vi "CurlingRobotforSweepHOST.vi"() -> ()   [LabVIEW 2015]
uses:
  <vilib>/IEDriver/SPIandI2C/Host/I2C/I2C Host.lvlib
  <vilib>/rvi/interface/nirviCloseFPGA/nirviCloseFPGA.xnode
  <vilib>/rvi/interface/nirviOpenFPGA/nirviOpenFPGA.xnode
  <vilib>/Platform/TimedLoop/XDataNode/wakeup.ctl
  <vilib>/Platform/TimedLoop/XDataNode/XDNodeRunTimeDep.lvlib
  <vilib>/Platform/TimedLoop/XDataNode/nitl_modes.ctl
  <vilib>/Platform/TimedLoop/XDataNode/timing_clust.ctl
  <vilib>/Platform/TimedLoop/XDataNode/XDataNode.xnode
  <vilib>/rvi/interface/nirviReadWriteControl/nirviReadWriteControl.xnode
  <vilib>/rvi/errors/niLvFpgaAdjustHostInterfaceError.vi
  <vilib>/rvi/interface/Simulation/niFpgaSimulationCallBeginRW.vi
  <vilib>/Instr/_visa.llb/VISA Flush IO Buffer Mask.ctl
  <vilib>/rvi/interface/nirviMethod/nirviMethod.xnode
  <vilib>/FPGAPlugInAG/Dynamic/niLvFpga_Reset_Dynamic.vi
  <vilib>/FPGAPlugInAG/Dynamic/niLvFpga_Run_Dynamic.vi
  cRIO_sweeping/SBC/Labview_exp/cRIO_sweeping/FPGA Bitfiles/testcomm_FPGATarget_FPGAsweepingaccg_gPSmUup16AQ.lvbitx
  cRIO_sweeping/SBC/Labview_exp/cRIO_sweeping/FPGA_sweeping_acc_gyro_v2.vi
  <vilib>/FPGAPlugInAG/cRIO-9033/niLvFpga_Open_cRIO-9033.vi
  <vilib>/rvi/interface/common/dynamic/niFpgaDynamicAddResources.vi
  NiFpgaLv.dll
  <vilib>/Utility/error.llb/Error Cluster From Error Code.vi
  <vilib>/FPGAPlugInAG/Dynamic/niLvFpga_Close_Dynamic.vi
  <vilib>/Instr/_visa.llb/VISA Configure Serial Port (Instr).vi
panel:
  in  "AddStAng":dbl=-7.0
  in  "FileCreat":bool
  out "AutobackCmd":i16(graph)
  in  "yStop":dbl=0.3 format="%#_13g"
  in  "upperx":dbl=0.3
  in  "downx":dbl=0.1 format="%#_13g"
  in  "LImitX":dbl=0.3 format="%#_13g"
  out "SBCAutoback":dbl
  out "NowVel13":dbl=-4.456150742348873e-97
  out "Steer_Rear":dbl=2.887351226806641
  out "RearSteerCmd":dbl
  out "CompleteAutoback":bool
  out "AutobackVel":dbl
  out "AutobackOn":bool
  out "Tqoff_autoback":bool=TRUE
  out "Time_autoback":dbl
  out "SBCvariable":dbl(graph)=2.0
  out "SBC2mode":bool
  out "sum_y":dbl=-7.853981633974483e-05
  out "sum_x":dbl
  out "Steer_Left":dbl=2.190110778808594
  out "OldAng":dbl
  out "SinTx":dbl
  in  "TxHz":dbl=50.0
  out "VelRef":dbl
  out "AutoTimer":dbl=13.18
  out "SBCmode 2":dbl(graph)=2.0
  out "AngRer":dbl
  in  "file create":bool
  out "File create":i32=1
  in  "Stop Button":bool
  out "Numeric Control":i32
  in  "data iner":bool
  out "data innter":i32=60895
  out "SBCAngReset":bool
  in  "DriveStart":bool
  out "Timing":u32(graph)=1
  out "loopTime":u32=1
  out "Yawrate":dbl(graph)
  in  "TqOn(On)":bool=TRUE
  in  "VelRef_0(off)":bool
  out "SBCEncReset":bool
  out "NowAng":dbl=70.04209333359984
  out "Tq_cmd_Rear":dbl=25.392464820602626
  in  "AngRef_0(off)":bool
  out "Read Data 2":string="10 ,     286.690948   1 , 0, 0, \r\n"
  in  "0.1V/deg":dbl=0.105
  in  "SetSteer":bool
  in  "90/10\nRealAng":dbl=1.0
  in  "정지":bool
  out "send":i32=61118
  out "TCPRecieve":i32=58477
  in  "Ang_ref\n1v=10deg":dbl(slide)=-24.97797356828194 scale=-90.0..90.0
  in  "SBCOn":bool=TRUE
  in  "V_target":dbl(slide)=0.07826086956521738 scale=-3.0..3.0
  out "DOBOnSBC":bool
  out "AskSBC4ABS":bool
  out "AskSBC":i16
  out "SBCSteerEnable":bool=TRUE
  out "CompliteABS":bool
  out "SBCDriveEnable":bool
  in  "Stop 2":bool
  out "send2SBC1":i16
  out "send2SBC 2":dbl
  out "send2SBC 3":dbl=-7.853981633974483e-05
  out "send2SBC 4":dbl=-4.456150742348873e-97
  in  "SendDataOn":bool
  in  "AbsErrorCrit":dbl=0.1
  out "SetSteer2Ori(On)":bool=TRUE
  in  "Steer3OriAbs 3":dbl=242.0
  out "Steer3NowAbs":dbl
  in  "Steer2OriAbs 2":dbl=242.133
  out "Steer2NowAbs":dbl
  out "Steer1NowAbs 2":dbl
  in  "Steer1OriAbs":dbl=242.051
  out "AngCmdDOB":dbl=-0.0
  out "RearAngCmd":dbl=25.392464820602626
  in  "AngReset2nowAng":bool
  in  "PhiAngCUT":dbl=2.0 format="%#_13g"
  in  "NowConfigAngle":dbl
  out "bias per 0.5min":dbl=-0.05348200000000247
  out "YawAngFB":dbl=289.95791201460014
  in  "RearTqScale":dbl=0.8
  out "YR_FB":dbl
  out "Tq_cmd_L":dbl=25.406420183499797
  out "Tq_cmd_R":dbl=25.397816125171232
  out "Yawangle":dbl=286.690948
  out "steering 2":T1(graph)={"Steer_Left"=2.190110778808594, "Steer_Right"=2.457696533203125, "Steer_Rear"=2.887351226806641, "Steer_ang_ref[NoScale] "=0.0}
  out "Velocity":cluster{"V_target":dbl, "Vel_Robot":dbl}(graph)={"V_target"=0.0, "Vel_Robot"=-4.456150742348873e-97}
  in  "Kt_longi":dbl=0.12
  out "Steer_ang_ref[NoScale]":dbl
  out "Vel_cmd":dbl
  out "x_Rear":dbl=-7.853981633974483e-05
  out "x_L":dbl
  out "x_R":dbl=-2.617993877991494e-05
  in  "YR*_zero(off)":bool
  out "Yawangle*":dbl
  in  "PD_cut_rot 2":dbl=15.0
  in  "Kp_rot 3":dbl=0.0002
  in  "Kd_rot 4":dbl=7e-05
  out "Yaw angle":cluster{dbl, "y":dbl, "Yawangle*":dbl}(graph)={0.0, "y"=70.04209333359984, "Yawangle*"=0.0}
  out "Driving_Left":i64
  in  "탭 컨트롤":T2(tab)=enum."Communication"
  out "Pmod_YR":dbl=-0.0009155413138017853
  out "acc 3":cluster{i16, i16, i16}(graph)={-1, 1, 229}
  in  "Timeout (10 s) 3":u8=50
  out "error out 5":errorcluster
  in  "Address 4":u16=29 format="%.0x"
  in  "Port Number 4":u8
  in  "FPGA Clock (40 MHz) 4":u32=40000000
  in  "Clock Rate 4":u32=100000 caption="Clock Rate"
  in  "Address Type (7-bit) 4":enum16{"7-bit", "10-bit"}(ring)
  in  "Address":u16=105 format="%.0x"
  in  "Port Number":u8=2
  in  "FPGA Clock (40 MHz)":u32=40000000
  in  "Clock Rate":u32=100000
  in  "Timeout (10 s)":u8=50
  in  "Address Type (7-bit)":enum16{"7-bit", "10-bit"}(ring)
  out "error out 3":errorcluster
  out "Pmod_acc_z":dbl=0.94824016563147
  out "Check_FPGA_Delay_loop":i32=22187
  out "Check":bool=TRUE
  out "Gyro sensors":cluster{"Pmod_YR":dbl, dbl, dbl, dbl, dbl}(graph)={"Pmod_YR"=-0.0009155413138017853, -0.0009054582550764345, -0.0009702831803661266, 5.4741866564341304e-05, 0.0}
  out "Time":i32=610853
  in  "ratelimit cut":dbl=30.0
  in  "yaw_ratelimit":dbl=5e-05
  in  "ratelimit band":dbl=0.0002
  out "Pmod_acc_x":dbl=-0.004140786749482402
  out "Pmod_acc_y":dbl=0.004140786749482402
  out "datameasure":i32=33453018
  out "writing":i32=51
  out "Degree":dbl(knob)=286.690948 scale=0.0..360.0
  out "Initalloop":i32=67261841
  out "error out":errorcluster caption="에러 출력"
  in  "error in":errorcluster caption="에러 입력"
  out "인덱스별 첫번째 바이트일 연속동기화횟수":u32[](array[numeric])=[7, 0, 0, 0]
  out "인덱스별 첫번째 바이트일 확률(%)":dbl[](array[numeric])=[100.0, 0.0, 0.0, 0.0] format="%.2f"
  out "초기 동기화 데이터 수신 횟수":i32=16
  out "초기 동기화 완료":bool
  out "error out 2":errorcluster caption="에러 출력"
  in  "error in 2":errorcluster caption="에러 입력"
  out "인덱스별 첫번째 바이트일 연속동기화횟수 2":u32[](array[numeric])=[724063, 0, 0, 0]
  out "인덱스별 첫번째 바이트일 확률(%) 2":dbl[](array[numeric])=[100.0, 0.0, 0.0, 0.0] format="%.2f"
  out "현재 동기화 완료":bool=TRUE
  out "최대 연속 동기화 횟수":u32=724063
  out "현재 데이터 수신 횟수":i32=724478
  out "Direction(CW-T, CCW-F)":bool=TRUE
  out "first subarray":bool[](array[boolean])=[TRUE, TRUE, TRUE, FALSE, FALSE, TRUE, TRUE, TRUE, FALSE, FALSE, TRUE, TRUE, TRUE, TRUE, FALSE, FALSE, TRUE, TRUE, TRUE, TRUE, TRUE, TRUE, TRUE]
  out "rawValue":i32=-49945
  out "Parity":bool
  out "Type":u32=2
  out "Synchronization":u32=2
  out "Message Validity":bool=TRUE
  out "동기화된 인덱스번호":u32[](array[numeric])=[2, 2, 2, 2, 2, 2, 2, 2, 2, 2, 2, 2, 2, 2]
  out "데이터오류횟수":i32=14
  out "버퍼된 문자개수":u32
  out "Yawangle 2":dbl=286.690948
  out "Wheel_Vel":T3(graph)={"y0"=1.0651839083712594e-105, "y0"=-4.91254963457663e-121, "y0"=-1.1967889933372377e-115, 1.0627795765209352e-84, -4.456150742348873e-97, -4.456150742348873e-97, "MinW"=-4.456150742348873e-97, "V_target"=0.0}
  in  "wheelV_ratelimit":dbl=0.001
  in  "Wheelvel_ratelimit cut":dbl=20.0
  out "Vel_Robot":dbl=-4.456150742348873e-97
  in  "Steeing_ang_limit":dbl=90.0
  in  "Steer_ang*_cut 2":dbl=0.5
  in  "Kp_wheelomega_Cont":dbl=1.8
  in  "right wheel FF_cut 2":dbl=8.0
  in  "J_FF_R_wh":dbl=0.001
  in  "B_FF_R_wh":dbl=4.0
  in  "Tqlim":dbl=4.0 format="%#_13g"
  out "SBCdata3":dbl
  out "SBCdata2":dbl
  out "SBCdata1":dbl
  out "SBCmode":dbl=2.0
  in  "port":u16=5100
  in  "address":string="192.168.1.105"
  in  "Kt_rot":dbl=0.126 format="%#_13g"
  in  "FF_cut":dbl=20.0
  in  "PD_cut_rot":dbl=20.0
  in  "Kp_rot 2":dbl=0.05
  in  "Kd_rot 3":dbl=0.005
  in  "J_FF_rot":dbl=0.1
  in  "B_FF_rot 2":dbl=0.05
  in  "YRContDOB":bool
  out "YMO FB":dbl=-0.0
  in  "DOB_FB_cut":dbl=20.0
  in  "Bm_rot":dbl=0.03
  in  "Jm_rot":dbl=0.02
  in  "Total_Stop":bool
  out "DeltaX":dbl(graph)
  in  "DrivingEnable":bool
  in  "SteerEnable":bool
  in  "DrvingEncReset":bool
  in  "Steer Enable":fxp<+/-,20,5>=10.0 format="%#_17g"
  in  "Driving Enable":fxp<+/-,20,5>=10.0 format="%#_17g"
  in  "SteerEncReset":bool
  in  "Driving_ENCVel_cut":dbl=25.0
  # "Yaw angle controller"
  # "Rot Velocity control with YMO"
  # "Auto back"
  # "Configuration"
  # "Write"
  # "1) Rate limiter"
  # "2) pickup most min vel among 3-wheels"
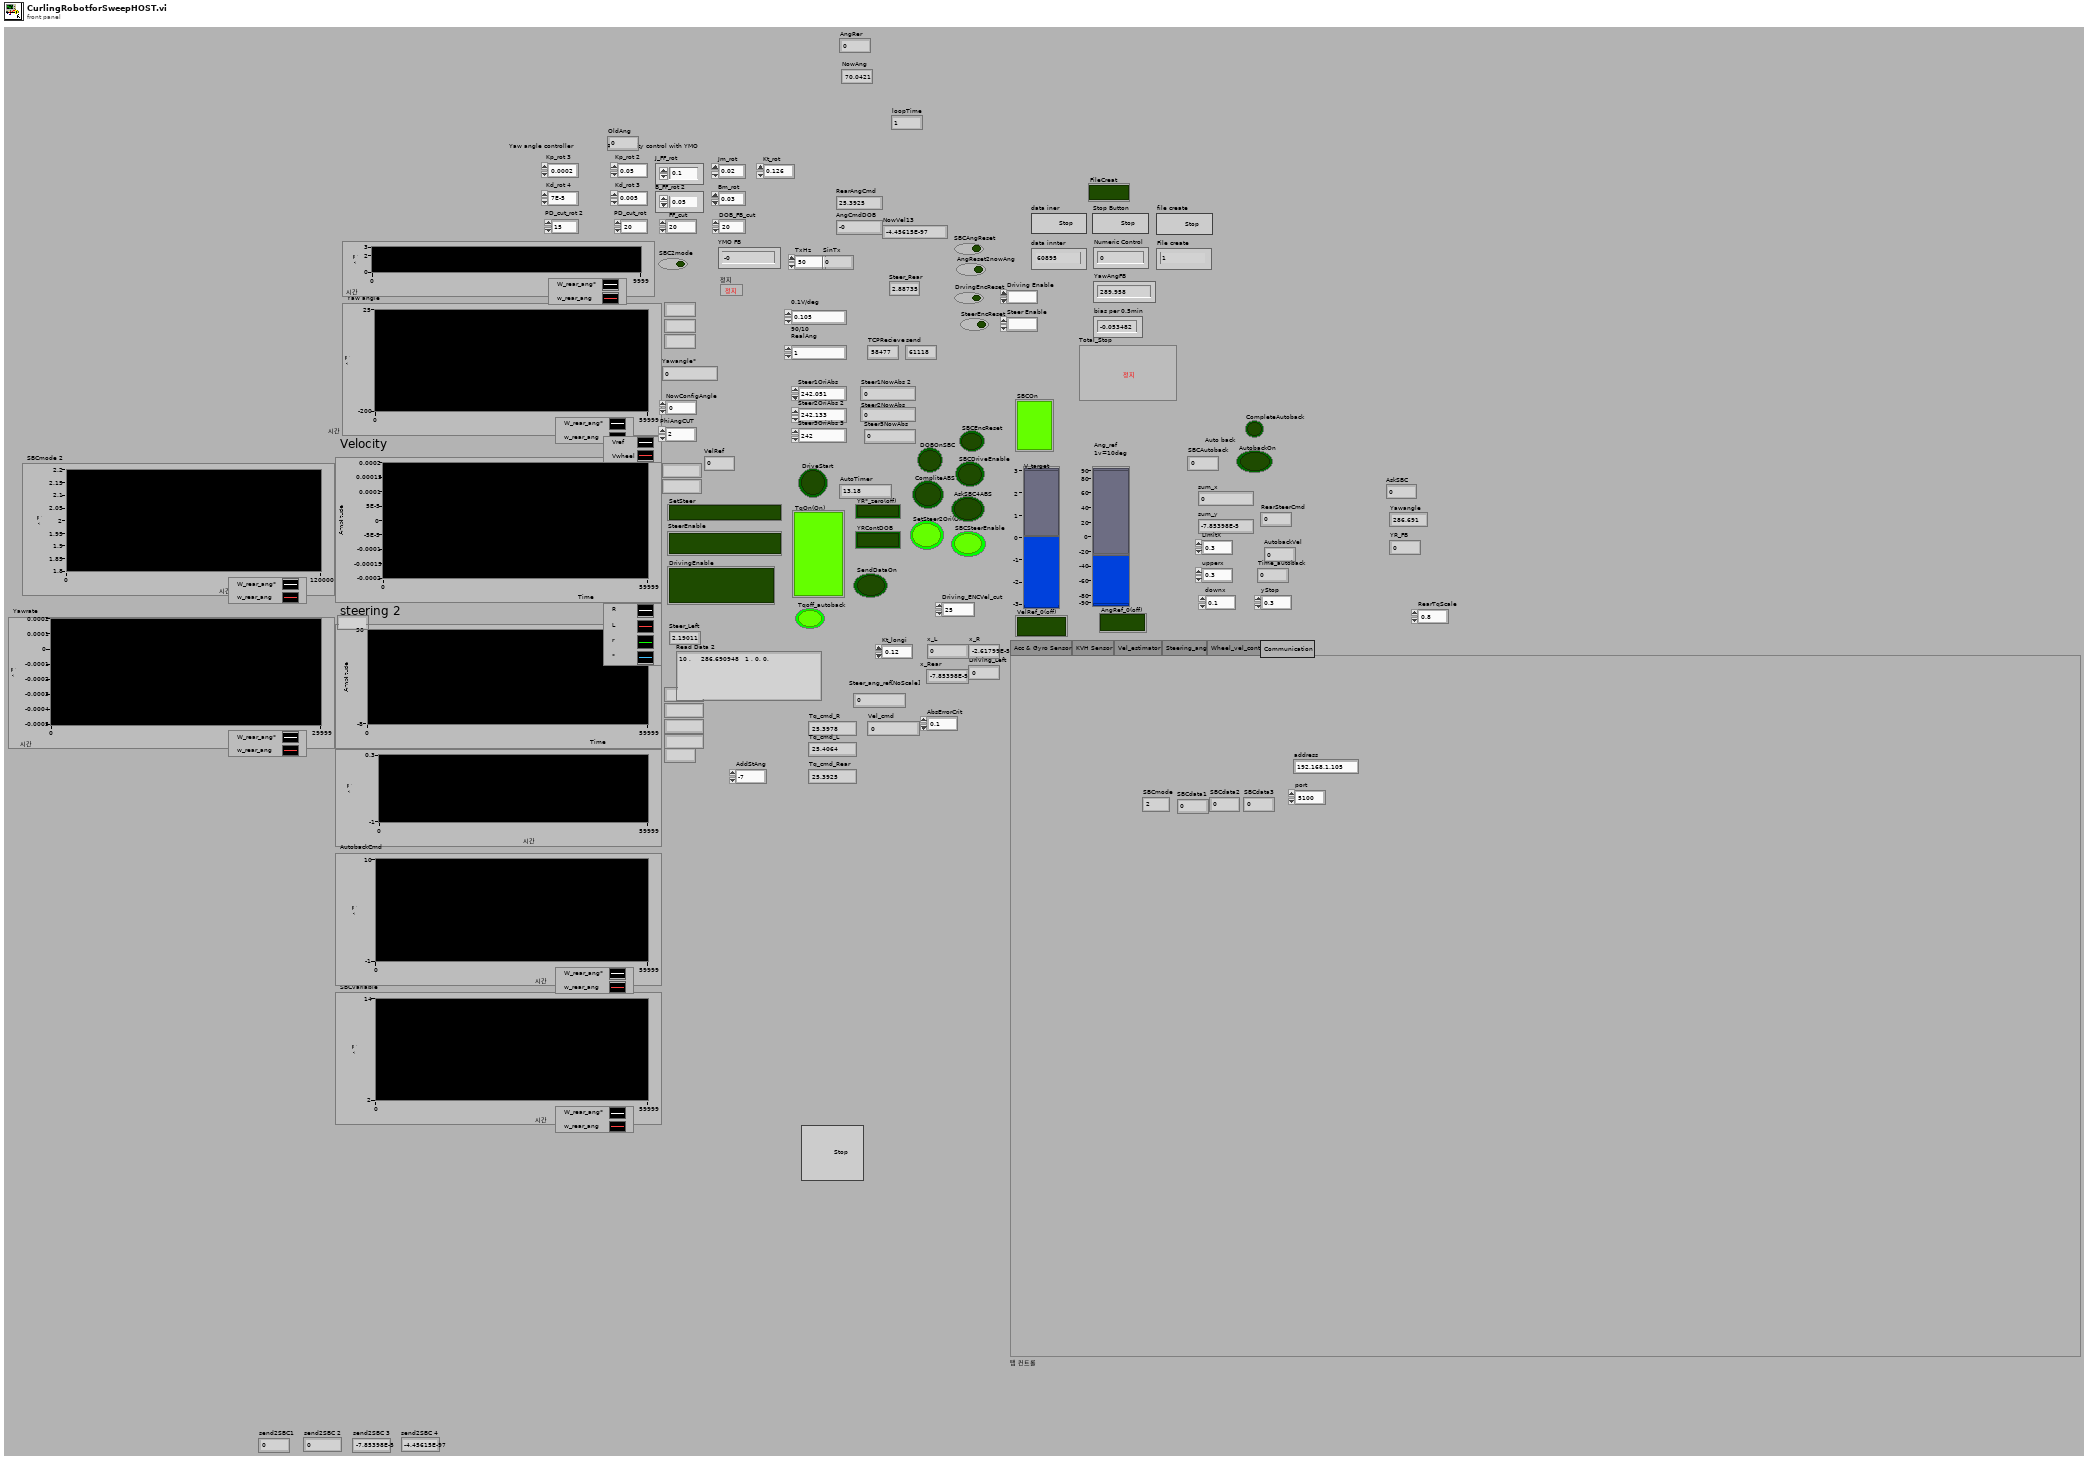
[diagram p1: front panel]
types:
  T1 = cluster{"Steer_Left":dbl, "Steer_Right":dbl, "Steer_Rear":dbl, "Steer_ang_ref[NoScale] ":dbl}
  T2 = enum32{"Acc & Gyro Sensor", "KVH Sensor", "Vel_estimator", "Steering_ang", "Wheel_vel_cont", "Communication"}
  T3 = cluster{"y0":dbl, "y0":dbl, "y0":dbl, dbl, dbl, dbl, "MinW":dbl, "V_target":dbl}
  T4 = typedef "VISA Flush IO Buffer Mask.ctl" = u16
  T5 = cluster{"baud rate":u32, "data bits":u16, "parity":enum16{"None", "Odd", "Even", "Mark", "Space"}, "stop bits":u16, "flow control":u16, "termination char":u8, "Enable Termination\nChar":bool, "timeout(ms)":u32}
  T6 = cluster{"FPGA VI Reference":refnum<k20>, "Port Number":u8}
  T7 = enum16{"Standard", "Buffered", "CRLF", "Immediate"}
  T8 = typedef "XDNodeRunTimeDep.lvlib/timing_clust.ctl" = cluster{"Expected End [f-1]":u64, "Actual End [f-1]":u64, "Finished Late? [f-1]":bool, "Expected End [i-1]":u64, "Actual End [i-1]":u64, "Finished Late? [i-1]":bool, "Expected Start [i]":u64, "Actual Start [i]":u64, "Expected Start [f]":u64, "Actual Start [f]":u64, "Source Name":string, "Structure Name":string, "Period":i64, "Deadline":i64, "Offset":i64, "Start":i64, "Priority":i32, "Timeout":i32, "Mode":T9, "Wakeup Reason":T10, "Error":errorcluster, "Source Type":string, "Secondary Source Type":string, "Global End Time":u64, "Global Start Time":u64, "Frame Duration":u64, "Iteration Duration":u64, "Assigned CPU":i32, "I/O Scan Engine Mode":u32}
  T9 = typedef "XDNodeRunTimeDep.lvlib/nitl_modes.ctl" = enum32{"No Change", "Process missed periods, maintain original phase", "Discard missed periods, maintain original phase", "Process missed periods, ignore original phase", "Discard missed periods, ignore original phase"}
  T10 = typedef "XDNodeRunTimeDep.lvlib/wakeup.ctl" = enum32{"Normal", "Aborted", "Asynchronous wakeup", "Timing source error", "Timed loop error", "Timeout"}
  T11 = cluster{"Steer_Left":i64, "Steer_Right":i64, "Steer_Rear":i64}
  T12 = cluster{"Steer_Left":dbl, "Steer_Right":dbl, "Steer_Rear":dbl}
  T13 = cluster{"Steer_Left":dbl, "Steer_Right":dbl, "Steer_Rear":dbl, "RearSteerCmd":dbl}
  T14 = cluster{"y0":dbl, "y0":dbl, "y0":dbl, dbl, dbl, dbl, "MinW":dbl, "f":dbl}
  T15 = enum16{"open", "replace", "create", "open or create", "replace or create", "replace or create with confirmation"}
  T16 = cluster{"x_L":dbl, "x_R":dbl, "x_Rear":dbl, "Vel_Robot":dbl, "VelRef":dbl, "AngRer":dbl, "NowAng":dbl, dbl, "SBCmode":dbl, "SinTx":dbl, "Jm_rot":dbl, dbl, "SBCmode 2":dbl}
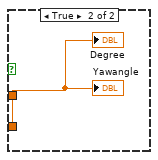
[diagram p4: hidden frame]
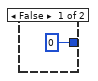
[diagram p9: hidden frame]
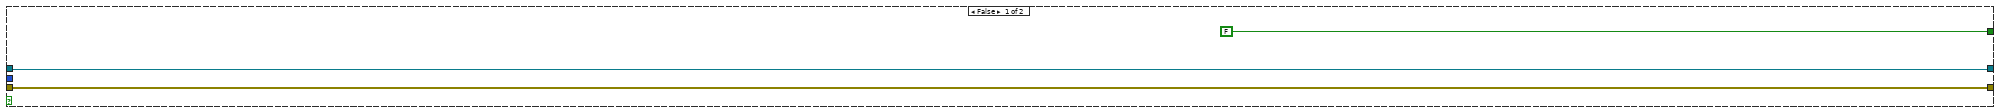
[diagram p12: hidden frame]
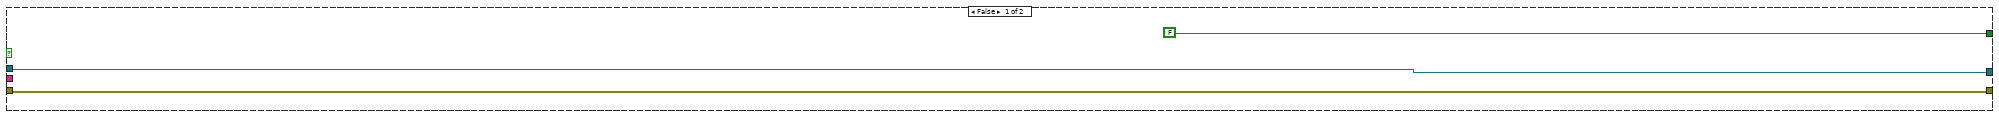
[diagram p13: hidden frame]
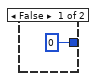
[diagram p14: hidden frame]
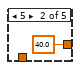
[diagram p20: hidden frame]
diagram:
  w22 = T4 16 items=["Flush Receive Buffer"=16, "Write Transmit Buffer to Device"=32, "Flush Receive Buffer (No I/O)"=64, "Flush Transmit Buffer"=128] ("Mask")
  w13 = T5 {"baud rate"=115200, "data bits"=8, "parity"=enum."None", "stop bits"=10, "flow control"=0, "termination char"=0, "Enable Termination\nChar"=FALSE, "timeout(ms)"=10000}  # VISA Configuration
  w12 = refnum<visa-resource-name> "ASRL1::INSTR"  # VISA resource name in
  # "DATA_READY to INT1, SINGLE_TAP to INT2"
  # "INT_MAP"
  # "Enable X-axis taps"
  # "TAP_AXES"
  # "Initialize device"
  # "Enable measurements"
  # "Enable DATA_READY and SINGLE_TAP interrupts"
  # "Duration = 10 ms"
  # "Tap threshold = 3g"
  # "POWER_CTL"
  # "INT_ENABLE"
  # "DUR"
  # "THRESH_TAP"
  # "Enable INT1 & \"data ready\" interrupt on INT2 pin"
  # "CTRL_REG3"
  # "Select HPF cutoff frequency"
  # "CTRL_REG2"
  # "Output select for LPF/HPF (both bypassed)"
  # "CTRL_REG5"
  # "Select data rate and enable measurements"
  # "Z-axis HI threshold"
  # "Enable interrupt on Z greater than HI threshold"
  # "CTRL_REG1"
  # "INT1_THS_ZH"
  # "INT1_CFG"
  # "Full scale setting = 100 dps"
  # "CTRL_REG4"
  # "register / data"
  # "4"
  # "3"
  # "2"
  # "1"
  n1 = Unbundle By Name(w13) -> ("Enable Termination\nChar"=w14:bool, "termination char"=w15:u8, "timeout(ms)"=w16:u32, "baud rate"=w21:u32, "data bits"=w20:u16, "parity"=w19:enum16{"None", "Odd", "Even", "Mark", "Space"}, "stop bits"=w18:u16, "flow control"=w17:u16)
  n2 = call-poly "VISA Configure Serial Port"("VISA resource name"=w12, "timeout (10sec)"=w16, "termination char\n(0xA = '\\n' = LF)"=w15, "Enable Termination\nChar (T)"=w14, "baud rate (9600)"=w21, "data bits (8)"=w20, "parity (0:none)"=w19, "error in (no error)"=w7, "stop bits (10: 1 bit)"=w18, "flow control (0:none)"=w17) -> ("VISA resource name out"=w11:refnum<visa-resource-name>, "error out"=w10:errorcluster)  [unwired: 4 in]
  n3 = VISA Flush I/O Buffer(VISA resource name=w11, mask (16)=w22, error in (no error)=w10) -> (VISA resource name out=w9:refnum<visa-resource-name>, error out=w8:errorcluster)
  n4 = flat-sequence {
    tunnel: [w56] -> w24
    tunnel: [w57] -> w23
    tunnel: [w65] -> w7
    tunnel: [w67] -> w31
    tunnel: w24 -> [w66]
    tunnel: w23 -> [w64]
    frame #0 {
      n5 = local write "Total_Stop"(FALSE ("정지")) -> ()
      n6 = xnode "FPGA VI 참조 열기"("리소스 이름"=tag "RIO0") -> ("FPGA VI 참조 출력"=w61:refnum<k20>, "에러 출력"=w60:errorcluster)  [unwired: 1 in]
      n7 = xnode "Invoke Method"("FPGA VI 참조 입력"=w61, "에러 입력"=w60) -> ("FPGA VI 참조 출력"=w58:refnum<k20>, "에러 출력"=w59:errorcluster)
      n8 = xnode "Invoke Method"("FPGA VI 참조 입력"=w58, "에러 입력"=w59, "완료될 때까지 기다림(거짓)"=FALSE) -> ("FPGA VI 참조 출력"=w56:refnum<k20>, "에러 출력"=w57:errorcluster)
      n9 = local write "SBCAutoback"(0.0 ("SBCAutoback")) -> ()
      n10 = local write "SBCmode"(2.0 ("SBCmode")) -> ()
    }
    frame #1 {
      n11 = while {
        tunnel: [w77] -> w67
        tunnel: w66 -> [w75]
        tunnel: [w76] -> w65
        tunnel: w64 -> [w78]
        i -> [w74]
        stop <- w68 stop-if-true
        w71 = 1000000 ("y")
        n12 = xnode "읽기/쓰기 컨트롤"("FPGA VI 참조 입력"=w75, "에러 입력"=w78) -> ("FPGA VI 참조 출력"=w77:refnum<k20>, "에러 출력"=w76:errorcluster, "FPGA_I2C_port0"=w73:i32, "FPGA_I2C_port2"=w72:i32)
        n13 = Greater?(x=w72, y=w71) -> (0:w69:bool)
        n14 = Greater?(x=w73, y=w71) -> (0:w70:bool)
        n15 = And(x=w70, y=w69) -> (x .and. y?=w68:bool)
        "Check" <- w68
        "Check_FPGA_Delay_loop" <- w74
      }
    }
  }
  n16 = while {
    tunnel: w8 -> [w82]
    tunnel: [w80] -> w5
    tunnel: w9 -> [w83]
    tunnel: [w89] -> w6
    i -> [w79]
    stop <- w88 stop-if-true
    w85 = u32 4 ("바이트 카운트")
    n17 = property class="Instr"(reference=w83, error in=w82) -> (reference out=w86:refnum<visa-resource-name>, error out=w81:errorcluster, "Serial Settings:Number of Bytes at Serial Port"=w87:u32)
    n18 = Greater Or Equal?(x=w87, y=w85) -> (x >= y?=w84:bool)
    n19 = case shown="참" w84 {
      tunnel: [w92 w102] -> w89
      tunnel: [FALSE ("동기화완료") w101] -> w88
      tunnel: w86 -> [w92 w100]
      tunnel: w85 -> [_ w93]
      tunnel: w81 -> [w90 w96]
      tunnel: [w90 w94] -> w80
      frame False {
      }
      frame True {
        # "데이터 수신 동기화"
        n20 = VISA Read(VISA resource name=w100, byte count=w93, error in (no error)=w96) -> (VISA resource name out=w97:refnum<visa-resource-name>, read buffer=w98:string, return count=w99:u32, error out=w95:errorcluster)
        n21 = Equal?(x=w99, y=w93) -> (x = y?=w103:bool)
        n22 = case shown="참" w103 {
          tunnel: w98 -> [_ w110]
          tunnel: w97 -> [w106 w127]
          tunnel: [w106 w126] -> w102
          tunnel: [FALSE w108] -> w101
          tunnel: w95 -> [w104 w122]
          tunnel: [w104 w121] -> w94
          frame False {
          }
          frame True {
            n23 = flat-sequence {
              tunnel: w110 -> [w130]
              tunnel: [w128] -> w120
              tunnel: w120 -> [w140]
              tunnel: [w141] -> w119
              tunnel: [w154] -> w118
              tunnel: [w153] -> w117
              tunnel: w119 -> [w152]
              tunnel: [w149] -> w116
              tunnel: [w148] -> w115
              tunnel: w118 -> [w165]
              tunnel: [w165] -> w114
              tunnel: w117 -> [w164]
              tunnel: [w164] -> w113
              tunnel: w116 -> [w162]
              tunnel: w115 -> [w161]
              tunnel: w114 -> [w176]
              tunnel: w113 -> [w174]
              tunnel: [w178] -> w109
              tunnel: [w174] -> w112
              tunnel: [w173] -> w108
              frame #0 {
                # "동기화 비트 추출"
                n24 = String To Byte Array(string=w130) -> (unsigned byte array=w129:u8[])
                n25 = for {
                  tunnel: w129 -> [w136] mode=indexing
                  tunnel: [w132] -> w128 mode=indexing
                  w134 = 2  # 할당비트 수
                  w135 = 5  # 동기화비트 인덱스
                  n26 = Number To Boolean Array(number=w136) -> (Boolean array=w131:bool[])
                  n27 = Array Subset(array=w131, index=w135, length=w134) -> (w133:bool[])
                  n28 = Boolean Array To Number(Boolean array=w133) -> (number=w132:u32)
                }
              }
              frame #1 {
                # "이전 동기화비트와 현재 동기화비트를 비교함\n이전 동기화비트에서 1을 더하여 현재와 비교함\n(동기화비트 3에서 1을 더할 경우\n4가 되므로 오류가 일어남 그래서\n동기화비트를 0으로 만듬)"
                n29 = feedback #1(w140) -> (w139:u32[])
                n30 = Increment(x=w139) -> (x+1=w138:u32[])
                n31 = feedback-in #1(w140) -> ()
                n32 = for {
                  tunnel: [w146] -> w137 mode=indexing
                  tunnel: w138 -> [w143] mode=indexing
                  n33 = Greater?(x=w143, y=u32 3 ("t")) -> (0:w144:bool)
                  n34 = Select(t=u32 0, s=w144, f=w143) -> (s? t:f=w146:u32)
                }
                n35 = Equal?(x=w140, y=w137) -> (x = y?=w141:bool[])
              }
              frame #2 {
                n36 = feedback #2(u32[] [0, 0, 0, 0]) -> (w150:u32[])
                n37 = for {
                  tunnel: w150 -> [w156] mode=indexing
                  tunnel: [w157] -> w149 mode=indexing
                  tunnel: w152 -> [w155] mode=indexing
                  # "동기화비트가 연속일 경우\n연속동기화회수를 증가"
                  n38 = case shown="참" w155 {
                    tunnel: [u32 0 w159] -> w157
                    tunnel: w156 -> [_ w160]
                    frame False {
                    }
                    frame True {
                      n39 = Increment(x=w160) -> (x+1=w159:u32)
                    }
                  }
                }
                "인덱스별 첫번째 바이트일 연속동기화횟수" <- w149
                n40 = feedback-in #2(w149) -> ()
                n41 = Array Max & Min(array=w149) -> (max value=w148:u32, max index (indices)=w153:i32)  [unwired: 2 out]
                n42 = Greater Or Equal?(x=w148, y=u32 7) -> (x >= y?=w154:bool)
              }
              frame #3 {
                n43 = for {
                  tunnel: w162 -> [w172] mode=indexing
                  tunnel: w161 -> [w171]
                  tunnel: [w166] -> w163 mode=indexing
                  w167 = 100.0  # %
                  n44 = To Double Precision Float(number=w172) -> (double precision float=w170:dbl)
                  n45 = To Double Precision Float(number=w171) -> (double precision float=w169:dbl)
                  n46 = Divide(x=w170, y=w169) -> (x/y=w168:dbl)
                  n47 = Multiply(x=w168, y=w167) -> (x*y=w166:dbl)
                }
                "인덱스별 첫번째 바이트일 확률(%)" <- w163
              }
              frame #4 {
                n48 = Equal To 0?(x=w174) -> (x = 0?=w175:bool)
                n49 = Compound Arithmetic op=AND ("복합 연산")(w176, w175) -> (w173:bool)
                n50 = Not Equal To 0?(x=w174) -> (x != 0?=w177:bool)
                n51 = Compound Arithmetic op=AND ("복합 연산")(w176, w177) -> (w178:bool)
              }
            }
            n52 = feedback #3(0) -> (w125:i32)
            n53 = Increment(x=w125) -> (x+1=w123:i32)
            "초기 동기화 데이터 수신 횟수" <- w123
            n54 = feedback-in #3(w123) -> ()
            n55 = To Unsigned Long Integer(number=w112) -> (unsigned 32bit integer=w107:u32)
            n56 = case shown="참" w109 {
              tunnel: w127 -> [w180 w185]
              tunnel: [w180 w184] -> w126
              tunnel: w107 -> [_ w183]
              tunnel: w122 -> [w179 w182]
              tunnel: [w179 w181] -> w121
              frame False {
              }
              frame True {
                n57 = VISA Read(VISA resource name=w185, byte count=w183, error in (no error)=w182) -> (VISA resource name out=w184:refnum<visa-resource-name>, error out=w181:errorcluster)  [unwired: 2 out]
              }
            }
            "error out" <- "error in"
          }
        }
      }
    }
    "초기 동기화 완료" <- w88
    "Initalloop" <- w79
  }
  n58 = TCP Open Connection(address="address", remote port or service name="port") -> (connection ID=w3:refnum<k5>, error out=w4:errorcluster)  [unwired: 3 in]
  n59 = call <vilib>:"I2C Configure.vi"("FPGA VI Reference"=w31, "Clock Rate"="Clock Rate", "Address"="Address", "Address Type (7-bit)"="Address Type (7-bit)", "Port Number"="Port Number", "error in (no error)"=w7, "FPGA Clock (40 MHz)"="FPGA Clock (40 MHz)") -> ("FPGA Information Out"=w44:T6, "error out"=w43:errorcluster)  [unwired: 7 in]
  n60 = while {
    tunnel: w4 -> [w191]
    tunnel: w3 -> [w190]
    i -> [w189]
    stop <- "정지" stop-if-true
    n61 = case shown="참" "SendDataOn" {
      tunnel: w190 -> [_ w204]
      tunnel: w191 -> [_ w192]
      frame False {
      }
      frame True {
        n62 = local read "send2SBC 2"() -> (w196:dbl)
        n63 = local read "send2SBC1"() -> (w193:i16)
        n64 = local read "send2SBC 4"() -> (w194:dbl)
        n65 = local read "send2SBC 3"() -> (w195:dbl)
        n66 = Format Value(value (0)=w193) -> (output string=w200:string)  [unwired: 2 in]
        n67 = Format Value(value (0)=w196) -> (output string=w199:string)  [unwired: 2 in]
        n68 = Format Value(value (0)=w195) -> (output string=w197:string)  [unwired: 2 in]
        n69 = Format Value(value (0)=w194) -> (output string=w198:string)  [unwired: 2 in]
        n70 = Format Into String(format string="%s,%s,%s,%s,XX" ("포맷 문자열"), w200, w199, w197, w198) -> (resulting string=w201:string)  [unwired: 2 in, 1 out]
        n71 = TCP Write(connection ID=w204, data in=w201, error in (no error)=w192, 9:-1 ("타임아웃 ms (25000)")) -> ()  [unwired: 3 out]
      }
    }
    n72 = Wait Until Next ms Multiple(millisecond multiple=u32 10 ("ms 배수")) -> ()  [unwired: 1 out]
    "send" <- w189
  }
  n73 = while {
    tunnel: w4 -> [w208]
    tunnel: w3 -> [w209]
    i -> [w206]
    stop <- "Stop 2" stop-if-true
    # "MOD가 GET 일 때만 TCP Read 하여 \n데이터 수신"
    # "TCP Client Loop"
    n74 = case shown="참" TRUE {
      tunnel: w209 -> [_ w217]
      tunnel: w208 -> [_ w216]
      frame False {
      }
      frame True {
        w229 = 512  # 읽을 바이트
        # "mode2, angle1, angle2, angle3"
        # "mode1, Steer1, Steer2, Steer3"
        # "mode4(stop), 0,0,0 ?"
        # "mode3, Vel_ref, beta, orient"
        n75 = TCP Read(connection ID=w217, bytes to read=w229, error in (no error)=w216, 7:T7."CRLF" ("모드(standard)"), 9:-1 ("타임아웃 ms (25000)")) -> (data out=w225:string)  [unwired: 2 out]
        "Read Data 2" <- w225
        n76 = Scan From String(format string="%s ,%s ,%s ,%s ,XX" ("포맷 문자열"), input string=w225) -> (output 1=w227:string, output 2=w223:string, output 3=w221:string, output 4=w219:string)  [unwired: 6 in, 3 out]
        n77 = Fract/Exp String To Number(string=w223, default (0 dbl)=0.0 ("default (0 DBL)")) -> (number=w213:dbl)  [unwired: 2 in, 1 out]
        n78 = Fract/Exp String To Number(string=w227, default (0 dbl)=0.0 ("default (0 DBL)")) -> (number=w210:dbl)  [unwired: 2 in, 1 out]
        n79 = Fract/Exp String To Number(string=w221, default (0 dbl)=0.0 ("default (0 DBL)")) -> (number=w212:dbl)  [unwired: 2 in, 1 out]
        n80 = Fract/Exp String To Number(string=w219, default (0 dbl)=0.0 ("default (0 DBL)")) -> (number=w211:dbl)  [unwired: 2 in, 1 out]
        n81 = Equal?(x=w210, y=10.0) -> (x = y?=w214:bool)
        n82 = case shown="거짓" w214 {
          tunnel: w213 -> [w234 w235]
          tunnel: w212 -> [w233 _]
          tunnel: w211 -> [w232 _]
          tunnel: w210 -> [w231 _]
          frame False {
            "SBCdata1" <- w234
            "SBCdata2" <- w233
            "SBCdata3" <- w232
            "SBCmode" <- w231
          }
          frame True {
            "Yawangle" <- w235
            "Degree" <- w235
          }
        }
      }
    }
    "TCPRecieve" <- w206
  }
  n83 = for {
    shift-right: [w240] -> w46
    shift-left: w44 -> [w238]
    shift-right: [w239] -> w45
    shift-left: w43 -> [w237]
    tunnel: u8[][] [[34, 136], [35, 0], [48, 32], [54, 80], [36, 0], [33, 9], [32, 15]] ("Bytes to Write") -> [w236] mode=indexing
    n84 = call <vilib>:"I2C Write.vi"("FPGA Information In"=w238, "Data"=w236, "error in (no error)"=w237) -> ("FPGA Information Out"=w240:T6, "error out"=w239:errorcluster)  [unwired: 11 in]
  }
  n85 = call <vilib>:"I2C Configure.vi"("FPGA VI Reference"=w31, "Clock Rate"="Clock Rate 4", "Address"="Address 4", "Address Type (7-bit)"="Address Type (7-bit) 4", "Port Number"="Port Number 4", "error in (no error)"=w7, "FPGA Clock (40 MHz)"="FPGA Clock (40 MHz) 4") -> ("FPGA Information Out"=w39:T6, "error out"=w40:errorcluster)  [unwired: 7 in]
  n86 = for {
    shift-right: [w245] -> w33
    shift-left: w39 -> [w243]
    shift-right: [w244] -> w32
    shift-left: w40 -> [w242]
    tunnel: u8[][] [[44, 10], [49, 11], [29, 48], [33, 16], [42, 4], [47, 64], [46, 192], [45, 8]] ("Bytes to Write") -> [w241] mode=indexing
    n87 = call <vilib>:"I2C Write.vi"("FPGA Information In"=w243, "Data"=w241, "error in (no error)"=w242) -> ("FPGA Information Out"=w245:T6, "error out"=w244:errorcluster)  [unwired: 11 in]
  }
  n88 = while {
    tunnel: w46 -> [w273]
    shift-right: [w271] -> w26
    shift-left: w45 -> [w274]
    stop <- w272 stop-if-true
    w266 = u16 6 ("Number of Bytes to Read")
    n89 = call <vilib>:"I2C Write.vi"("FPGA Information In"=w273, "Data"=u8[] [168] ("Write Data"), "error in (no error)"=w274, "Timeout (10 s)"="Timeout (10 s)") -> ("FPGA Information Out"=w269:T6, "error out"=w270:errorcluster)  [unwired: 10 in]
    n90 = Initialize Array(u8 0, w266) -> (w264:u8[])
    n91 = call <vilib>:"I2C Read.vi"("FPGA Information In"=w269, "Input Array"=w264, "Number of Bytes to Read"=w266, "error in (no error)"=w270, "Timeout (10 s)"="Timeout (10 s)") -> ("Data"=w260:u8[], "error out"=w271:errorcluster)  [unwired: 8 in, 1 out]
    "error out 3" <- w271
    n92 = Index Array(array=w260) -> (element #1=w259:u8, element #2=w258:u8, element #3=w255:u8, element #4=w254:u8, element #5=w257:u8, element #6=w256:u8)  [unwired: 6 in]
    n93 = Join Numbers(hi=w258, lo=w259) -> ((hi.lo)=w263:u16)
    n94 = Join Numbers(hi=w254, lo=w255) -> ((hi.lo)=w262:u16)
    n95 = Join Numbers(hi=w256, lo=w257) -> ((hi.lo)=w261:u16)
    n96 = To Word Integer(number=w263) -> (16bit integer=w253:i16)
    n97 = To Word Integer(number=w262) -> (16bit integer=w252:i16)
    n98 = To Word Integer(number=w261) -> (16bit integer=w251:i16)
    n99 = Bundle "Bundle"(w253, w252, w251) -> (w250:cluster{i16, i16, i16})  [unwired: 1 in]
    n100 = local read "Total_Stop"() -> (w246:bool)
    n101 = Unbundle(w250) -> (w249:i16)  [unwired: 2 out]
    n102 = Divide(x=w249, y=65535.0) -> (x/y=→"Pmod_YR":dbl)
    n103 = Or(x=w271, y=w246) -> (x .or. y?=w272:bool)
  }
  n104 = while {
    tunnel: w6 -> [w281]
    tunnel: w5 -> [w280]
    tunnel: [w276] -> _
    tunnel: [w275] -> _
    i -> [w284]
    stop <- w277 stop-if-true
    w278 = 5.0  # y
    w294 = u32 10  # ms 배수
    n105 = Wait Until Next ms Multiple(millisecond multiple=w294) -> ()  [unwired: 1 out]
    n106 = Divide(x=w284, y=10) -> (x/y=w279:dbl)
    n107 = Greater?(x=w279, y=1.0) -> (0:w289:bool)
    n108 = Greater?(x=w279, y=3.0) -> (0:w286:bool)
    n109 = Less?(x=w279, y=2.0) -> (x < y?=w288:bool)
    n110 = Greater?(x=w279, y=w278) -> (0:w277:bool)
    n111 = Less?(x=w279, y=4.0) -> (x < y?=w285:bool)
    n112 = And(x=w286, y=w285) -> (x .and. y?=w282:bool)
    n113 = And(x=w289, y=w288) -> (x .and. y?=w283:bool)
    n114 = case shown="참" w283 {
      tunnel: w281 -> [_ w306]
      tunnel: w280 -> [w302 w305]
      tunnel: [w302 w304] -> w275
      frame False {
      }
      frame True {
        w303 = "Z"  # 명령 선택
        n115 = VISA Write(VISA resource name=w306, write buffer=w303, error in (no error)=w305) -> (error out=w304:errorcluster)  [unwired: 2 out]
      }
    }
    n116 = case shown="참" w282 {
      tunnel: w281 -> [w295 w301]
      tunnel: w280 -> [w296 w300]
      tunnel: [w296 w299] -> _
      tunnel: [w295 w297] -> w276
      frame False {
      }
      frame True {
        w298 = "P"  # 명령 선택
        n117 = VISA Write(VISA resource name=w301, write buffer=w298, error in (no error)=w300) -> (VISA resource name out=w297:refnum<visa-resource-name>, error out=w299:errorcluster)  [unwired: 1 out]
      }
    }
    "writing" <- w284
  }
  n118 = while {
    shift-right: [w335] -> w27
    shift-left: w32 -> [w352]
    tunnel: w33 -> [w320]
    stop <- w350 stop-if-true
    w333 = u16 6 ("Number of Bytes to Read")
    w345 = u16 1 ("Number of Bytes to Read")
    n119 = call <vilib>:"I2C Write.vi"("FPGA Information In"=w320, "Data"=u8[] [48] ("Write Data"), "error in (no error)"=w352, "Timeout (10 s)"="Timeout (10 s) 3") -> ("FPGA Information Out"=w348:T6, "error out"=w349:errorcluster)  [unwired: 10 in]
    n120 = Initialize Array(u8 0, w345) -> (w343:u8[])
    n121 = call <vilib>:"I2C Read.vi"("FPGA Information In"=w348, "Input Array"=w343, "Number of Bytes to Read"=w345, "error in (no error)"=w349, "Timeout (10 s)"="Timeout (10 s) 3") -> ("FPGA Information Out"=w341:T6, "error out"=w336:errorcluster)  [unwired: 8 in, 1 out]
    n122 = call <vilib>:"I2C Write.vi"("FPGA Information In"=w341, "Data"=u8[] [50] ("Write Data"), "error in (no error)"=w336) -> ("FPGA Information Out"=w338:T6, "error out"=w337:errorcluster)  [unwired: 11 in]
    n123 = Initialize Array(u8 0, w333) -> (w334:u8[])
    n124 = call <vilib>:"I2C Read.vi"("FPGA Information In"=w338, "Input Array"=w334, "Number of Bytes to Read"=w333, "error in (no error)"=w337) -> ("Data"=w323:u8[], "error out"=w335:errorcluster)  [unwired: 9 in, 1 out]
    "error out 5" <- w335
    n125 = Index Array "Index Array"(array=w323) -> (element #1=w329:u8, element #2=w328:u8, element #3=w327:u8, element #4=w326:u8, element #5=w325:u8, element #6=w324:u8)  [unwired: 6 in]
    n126 = Join Numbers(hi=w328, lo=w329) -> ((hi.lo)=w332:u16)
    n127 = Join Numbers(hi=w326, lo=w327) -> ((hi.lo)=w331:u16)
    n128 = Join Numbers(hi=w324, lo=w325) -> ((hi.lo)=w330:u16)
    n129 = To Word Integer(number=w332) -> (16bit integer=w316:i16)
    n130 = To Word Integer(number=w331) -> (16bit integer=w318:i16)
    n131 = To Word Integer(number=w330) -> (16bit integer=w321:i16)
    n132 = Bundle "Bundle"(w316, w318, w321) -> (→"acc 3":cluster{i16, i16, i16})  [unwired: 1 in]
    n133 = Divide(x=w321, y=1.0) -> (x/y=w308:dbl)
    n134 = Divide(x=w318, y=1.0) -> (x/y=w311:dbl)
    n135 = Or(x=w335, y="Total_Stop") -> (x .or. y?=w350:bool)
    n136 = Divide(x=w316, y=1.0) -> (x/y=w315:dbl)
    n137 = Divide(x=w308, y=241.5) -> (x/y=→"Pmod_acc_z":dbl)
    n138 = Divide(x=w311, y=241.5) -> (x/y=→"Pmod_acc_y":dbl)
    n139 = Divide(x=w315, y=241.5) -> (x/y=→"Pmod_acc_x":dbl)
  }
  n140 = node-c288() -> (w30:T8)  [unwired: 4 in]
  n141 = timed-loop {
    timing: w30 -> [_]
    timing-out: [_] -> w29
    tunnel: w31 -> [w1144]
    tunnel: w7 -> [w1007]
    i -> [w840]
    stop <- w1006 stop-if-true
    w831 = 0.0
    w853 = 0.0
    w1051 = 0.001 ("input variable")
    w1085 = 0.0
    w1140 = 0.0 ("y0")
    w1129 = 0.001 ("input variable")
    w1135 = 40000.0 ("y")
    w1136 = 6.283185307179586
    # "DATA Save"
    # "Because refsteer offset"
    # "Yaw LPF"
    # "within 0.1m"
    # "Driving Starting Timing To Sync for Throwing robot"
    # "Reset when ''2' input"
    # "Time only SBC1 is '7'"
    # "until"
    # "Configuration Controller"
    # "Send 2 SBC ABS complite(DrivingReady)"
    # "Rotate ABS  after get ABS"
    # "When power On get ABS and control"
    # "Send to SBC Communication"
    # "When ''4'' In, send SBC every 10ms and switch to 9"
    # "Always On"
    # "Power On after get ABS Rotate Steer ABS Start"
    # "When End driving get ABS"
    # "Phi Control input"
    # "Steering Ang Direct Input"
    # "Steering Ang Cmd"
    # "To get origine angle"
    # "YR_ref"
    # "phi_FB"
    # "angle limit +-180"
    # "KVH sensor bias remover"
    # "To remove 360.6~~"
    # "Right wheel FF"
    # "Right wheel FF"
    # "Right wheel FF"
    # "Wheel_omega"
    # "Steering part controller Steering part controller Steering part controller Steering part controller Steering part controller Steering part controller Steering part controller Steering part controller Steering part controller Steering part controller Steering part controller Steering part controller Steering part controller Steering part controller Steering part controller Steering part controller Steering part controller Steering part controller Steering part controller Steering part controller Steering part controller Steering part controller"
    # "rated limiter"
    # "rated limiter"
    # "rated limiter"
    # "Rbot velocity Estimation\n1) put in rate limit each wheel.\n2) pick up mim wheelvel among 3-wheel.\n3) KKF with acceleration"
    # "Yaw LPF"
    # "Rot PD  controller"
    # "yaw rate FF"
    # "Rot PD  controller"
    # "Mz in"
    # "Gyro FB"
    # "YMO controller"
    # "Gyrosensor offset remover"
    # "calculatefixed offset"
    # "Rate limiter"
    # "rated limiter"
    # "Steering Enc part(abs)"
    # "Driving Enc part"
    # "cnt/rev19bit"
    # "Simga"
    # "Rear is just semi-passive"
    # "Wheel_omega"
    # "Select manual Omega"
    # "Wheel velocity"
    # "Select manual Tq"
    # "Elmo In Saturation"
    # "W_L"
    # "W_B"
    # "W_R"
    # "Vw_PI controller 3wheels"
    # "T_R*"
    # "Time derivative of enc to gel wheel vel"
    # "Wheel encoder gear ratio, encoder"
    # "gear ratio"
    # "gear ratio"
    n142 = node-c288() -> ()  [unwired: 1 in, 1 out]
    n143 = local read "SBCEncReset"() -> (w556:bool)
    n144 = Or(x="SteerEncReset", y=w556) -> (x .or. y?=w613:bool)
    n145 = Or(x="DrvingEncReset", y=w556) -> (x .or. y?=w612:bool)
    n146 = xnode "읽기/쓰기 컨트롤"("FPGA VI 참조 입력"=w1144, "에러 입력"=w1007, "QuadENC2Reset 2"=w613, "QuadENC3Reset 5"=w613, "QuadENC3Reset 4"=w613, "QuadENC2Reset"=w612, "QuadENC3Reset 3"=w612, "QuadENC3Reset 2"=w612) -> ("FPGA VI 참조 출력"=w1146:refnum<k20>, "에러 출력"=w1145:errorcluster, "Driving_Left"=w1138:i64, "Driving_Right"=w1126:i64, "Driving_Rear"=w1137:i64, "Steer_Left"=w1114:i64, "Steer_Right"=w1113:i64, "Steer_Rear"=w1112:i64)
    "Driving_Left" <- w1138
    n147 = feedback #4(0.0 ("gy_ratelimit")) -> (w968:dbl)
    n148 = feedback #5(0.0 ("gy_ratelimit")) -> (w945:dbl)
    n149 = feedback #6(0.0) -> (w460:dbl)
    n150 = feedback #7(0.0 ("gy_ratelimit")) -> (w946:dbl)
    n151 = feedback #8(0.0) -> (w963:dbl)
    n152 = feedback #9(0.0) -> (w943:dbl)
    n153 = feedback #10(0.0) -> (w948:dbl)
    n154 = Multiply(x="Wheelvel_ratelimit cut", y=6.283185307179586) -> (x*y=w965:dbl)
    n155 = Reciprocal(x=w965) -> (1/x=w935:dbl)
    n156 = Multiply(x=1.0 ("PhiAngCUT 2"), y=6.283185307179586) -> (x*y=w464:dbl)
    n157 = Multiply(x=w1138, y=w1136) -> (x*y=w1165:dbl)
    n158 = Multiply(x=w1126, y=w1136) -> (x*y=w1164:dbl)
    n159 = Multiply(x=w1137, y=w1136) -> (x*y=w1134:dbl)
    n160 = Bundle("Steer_Left"=w1114, "Steer_Right"=w1113, "Steer_Rear"=w1112) -> (w1110:T11)  [unwired: 1 in]
    n161 = Reciprocal(x=w464) -> (1/x=w466:dbl)
    n162 = Multiply(x=w1110, y=6.283185307179586) -> (x*y=w1109:T12)
    n163 = Divide(x=w1109, y=524288.0) -> (x/y=w1106:T12)
    n164 = Divide(x=w1165, y=w1135) -> (x/y=w1130:dbl)
    n165 = Divide(x=w1164, y=w1135) -> (x/y=w1131:dbl)
    n166 = Divide(x=w1134, y=w1135) -> (x/y=w1132:dbl)
    n167 = local read "RearSteerCmd"() -> (w456:dbl)
    n168 = feedback-in #6(w456) -> ()
    n169 = Divide(x=w1106, y=100.0) -> (x/y=w655:T12)
    n170 = Multiply(x=w655, y=180.0) -> (x*y=w653:T12)
    n171 = Divide(x=w653, y=3.141592653589793) -> (x/y=w652:T12)
    n172 = feedback #11(0.0) -> (w1160:dbl)
    n173 = feedback-in #11(w1130) -> ()
    n174 = feedback #12(0.0) -> (w1143:dbl)
    n175 = feedback-in #12(w1131) -> ()
    n176 = feedback #13(0.0) -> (w1157:dbl)
    n177 = feedback-in #13(w1132) -> ()
    n178 = feedback #14(0.0) -> (w967:dbl)
    n179 = feedback #15(0.0) -> (w944:dbl)
    n180 = feedback #16(0.0) -> (w947:dbl)
    n181 = Bundle(w1131, w1130, w1132) -> (w1151:cluster{dbl, dbl, dbl})  [unwired: 1 in]
    n182 = local read "YawAngFB"() -> (w624:dbl)
    n183 = feedback #17(0.0) -> (w461:dbl)
    n184 = formula code="float F,A,B,C,y0;\nF=2*tau+T;\nA=(2*a+b*T)/F;\nB=(b*T-2*a)/F;\nC=(2*tau-T)/F;\ny0=A*u0+B*u1+C*y1;"("tau"=w466, "u0"=w456, "u1"=w460, "y1"=w461, "T"=0.001 ("입력 변수"), "a"=0.0 ("input variable"), "b"=1.0 ("input variable")) -> ("y0"=w457:dbl)
    n185 = feedback-in #17(w457) -> ()
    n186 = Multiply(x="Driving_ENCVel_cut", y=6.283185307179586) -> (x*y=w1162:dbl)
    n187 = Reciprocal(x=w1162) -> (1/x=w1133:dbl)
    n188 = Divide(x=w1151, y=6.0) -> (x/y=w1148:cluster{dbl, dbl, dbl})
    n189 = Multiply(x=w1148, y=0.125) -> (x*y=w918:cluster{dbl, dbl, dbl})
    n190 = local read "SBCAngReset"() -> (w559:bool)
    n191 = formula code="float phi;\nif (sensor > 180 && sensor <= 360)\nphi = sensor-360;\nelse\nphi = sensor;"("sensor"=w624) -> ("phi"=w837:dbl)
    n192 = Unbundle(w918) -> (→"x_R":dbl, →"x_L":dbl, →"x_Rear":dbl)
    n193 = local read "Yawangle"() -> (→"Yawangle 2":dbl)
    n194 = feedback #18(w1140) -> (w1158:dbl)
    n195 = formula code="y0=(2*(u0-u1)-(T-2*Tau)*y1)/(T+2*Tau);"("Tau"=w1133, "u0"=w1132, "u1"=w1157, "y1"=w1158, "T"=w1129) -> ("y0"=w1154:dbl)
    n196 = feedback-in #18(w1154) -> ()
    n197 = feedback #19(w1140) -> (w1161:dbl)
    n198 = formula code="y0=(2*(u0-u1)-(T-2*Tau)*y1)/(T+2*Tau);"("Tau"=w1133, "u0"=w1130, "u1"=w1160, "y1"=w1161, "T"=w1129) -> ("y0"=w1150:dbl)
    n199 = feedback-in #19(w1150) -> ()
    n200 = feedback #20(w1140) -> (w1141:dbl)
    n201 = formula code="y0=(2*(u0-u1)-(T-2*Tau)*y1)/(T+2*Tau);"("Tau"=w1133, "u0"=w1131, "u1"=w1143, "y1"=w1141, "T"=w1129) -> ("y0"=w1139:dbl)
    n202 = feedback-in #20(w1139) -> ()
    n203 = local read "Vel_cmd"() -> (w552:dbl)
    n204 = feedback #21(0.0) -> (w358:dbl)
    n205 = local read "SBCmode"() -> (w397:dbl)
    "SBCmode 2" <- w397
    n206 = Equal?(x=w397, y=13.0) -> (x = y?=w398:bool)
    n207 = local read "x_Rear"() -> (w531:dbl)
    n208 = Or(x=w559, y="AngReset2nowAng") -> (x .or. y?=w386:bool)
    n209 = case shown="참" w386 {
      frame False {
      }
      frame True {
        w1178 = 0.0 ("sum_x")
        n210 = local write "DeltaX"(w1178) -> ()
        n211 = local write "sum_x"(w1178) -> ()
        n212 = local write "sum_y"(w1178) -> ()
      }
    }
    n213 = Bundle("y0"=w1139, "y0"=w1150, "y0"=w1154) -> (w1149:cluster{"y0":dbl, "y0":dbl, "y0":dbl})  [unwired: 1 in]
    n214 = Negate(x=w837) -> (-x=w639:dbl)
    n215 = feedback #22(0.0) -> (w994:dbl)
    n216 = Divide(x=w1149, y=6.0) -> (x/y=w896:cluster{"y0":dbl, "y0":dbl, "y0":dbl})
    n217 = case shown="참" w398 {
      tunnel: w397 -> [_ w1170]
      frame False {
      }
      frame True {
        "SBCAutoback" <- w1170
      }
    }
    n218 = expression code="(x/180.0)*pi" "도를 라디안으로"(w457) -> (w528:dbl)
    n219 = local read "Yawangle*"() -> (w557:dbl)
    n220 = feedback #23(0.0 ("x_Rear")) -> (w530:dbl)
    n221 = feedback-in #23(w531) -> ()
    n222 = Multiply(x=w896, y=0.125 ("x")) -> (x*y=w920:cluster{"y0":dbl, "y0":dbl, "y0":dbl})
    n223 = Unbundle(w920) -> ("y0"=w932:dbl, "y0"=w933:dbl)  [unwired: 1 out]
    n224 = formula code="float rate;\nrate=gy-gy_r1;\nif (rate > limit)\ngy_ratelimit=gy_r1+limit;\nelse if (rate < -limit)\ngy_ratelimit=gy_r1+(-limit);\nelse\ngy_ratelimit=gy;"("gy"=w932, "gy_r1"=w968, "limit"="wheelV_ratelimit") -> ("gy_ratelimit"=w956:dbl)
    n225 = formula code="float rate;\nrate=gy-gy_r1;\nif (rate > limit)\ngy_ratelimit=gy_r1+limit;\nelse if (rate < -limit)\ngy_ratelimit=gy_r1+(-limit);\nelse\ngy_ratelimit=gy;"("gy"=w933, "gy_r1"=w945, "limit"="wheelV_ratelimit") -> ("gy_ratelimit"=w936:dbl)
    n226 = formula code="float rate;\nrate=gy-gy_r1;\nif (rate > limit)\ngy_ratelimit=gy_r1+limit;\nelse if (rate < -limit)\ngy_ratelimit=gy_r1+(-limit);\nelse\ngy_ratelimit=gy;"("gy"=w933, "gy_r1"=w946, "limit"="wheelV_ratelimit") -> ("gy_ratelimit"=w955:dbl)
    n227 = feedback-in #4(w956) -> ()
    n228 = feedback-in #5(w936) -> ()
    n229 = feedback-in #7(w955) -> ()
    n230 = feedback-in #8(w956) -> ()
    n231 = feedback-in #9(w936) -> ()
    n232 = feedback-in #10(w955) -> ()
    n233 = formula code="float F,A,B,C,y0;\nF=2*tau+T;\nA=(2*a+b*T)/F;\nB=(b*T-2*a)/F;\nC=(2*tau-T)/F;\ny0=A*u0+B*u1+C*y1;"("tau"=w935, "u0"=w956, "u1"=w963, "y1"=w967, "T"=0.001 ("input variable"), "a"=0.0 ("input variable"), "b"=1.0 ("input variable")) -> ("y0"=w931:dbl)
    n234 = formula code="float F,A,B,C,y0;\nF=2*tau+T;\nA=(2*a+b*T)/F;\nB=(b*T-2*a)/F;\nC=(2*tau-T)/F;\ny0=A*u0+B*u1+C*y1;"("tau"=w935, "u0"=w936, "u1"=w943, "y1"=w944, "T"=0.001 ("input variable"), "a"=0.0 ("input variable"), "b"=1.0 ("input variable")) -> ("y0"=w929:dbl)
    n235 = formula code="float F,A,B,C,y0;\nF=2*tau+T;\nA=(2*a+b*T)/F;\nB=(b*T-2*a)/F;\nC=(2*tau-T)/F;\ny0=A*u0+B*u1+C*y1;"("tau"=w935, "u0"=w955, "u1"=w948, "y1"=w947, "T"=0.001 ("input variable"), "a"=0.0 ("input variable"), "b"=1.0 ("input variable")) -> ("y0"=w930:dbl)
    n236 = feedback-in #14(w931) -> ()
    n237 = feedback-in #15(w929) -> ()
    n238 = feedback-in #16(w930) -> ()
    n239 = Bundle(w931, w930, w929) -> (w925:cluster{dbl, dbl, dbl})  [unwired: 1 in]
    n240 = formula code="float W12,W123;\nif (abs(W1) > abs(W2))\nW12=W2;\nelse\nW12=W1;\n\nif (abs(W12) > abs(W3))\nW123= W3;\nelse\nW123=W12;\n\nMinW=W123;"("W1"=w931, "W2"=w930, "W3"=w929) -> ("MinW"=w924:dbl)
    "Vel_Robot" <- w924
    n241 = Unbundle(w925) -> (w928:dbl, w927:dbl, w926:dbl)
    n242 = Unbundle(w920) -> ("y0"=w922:dbl, "y0"=w921:dbl, "y0"=w919:dbl)
    n243 = local read "Time"() -> (w577:i32)
    n244 = Multiply(x="PD_cut_rot 2", y=6.283185307179586) -> (x*y=w991:dbl)
    n245 = Reciprocal(x=w991) -> (1/x=w992:dbl)
    n246 = Unbundle(w896) -> ("y0"=w1115:dbl, "y0"=w1116:dbl, "y0"=w1120:dbl)
    n247 = Equal?(x=w397, y=10.0) -> (x = y?=w404:bool)
    n248 = local read "Steer_ang_ref[NoScale]"() -> (w354:dbl)
    n249 = Add(x="AddStAng", y=w354) -> (x+y=w355:dbl)
    n250 = Unbundle(w920) -> ("y0"=w1119:dbl, "y0"=w1118:dbl, "y0"=w1117:dbl)
    n251 = Subtract(x=w531, y=w530) -> (x-y=w527:dbl)
    n252 = case shown="거짓" w404 {
      tunnel: w397 -> [w1187 _]
      frame False {
        "SBCvariable" <- w1187
      }
      frame True {
      }
    }
    n253 = Bundle("y0"=w1115, "y0"=w1116, "y0"=w1120) -> ()  [unwired: 1 in, 1 out]
    n254 = local read "RearSteerCmd"() -> (w467:dbl)
    n255 = formula code="y=l*cos(th);\nx=l*sin(th);"("l"=w527, "th"=w528) -> ("x"=w526:dbl, "y"=w523:dbl)
    n256 = Bundle("y0"=w1119, "y0"=w1118, "y0"=w1117) -> ()  [unwired: 1 in, 1 out]
    n257 = Divide(x=w577, y=1000) -> (x/y=w576:dbl)
    n258 = Unbundle(w652) -> ("Steer_Left"=w658:dbl, "Steer_Right"=w659:dbl, "Steer_Rear"=w660:dbl)
    "Steer_Left" <- w658
    "Steer_Rear" <- w660
    n259 = Add(x=w557, y="NowConfigAngle") -> (x+y=w838:dbl)
    n260 = Bundle("Steer_Left"=w658, "Steer_Right"=w659, "Steer_Rear"=w660, "RearSteerCmd"=w467) -> (→"steering 2":T13)  [unwired: 1 in]
    n261 = local read "AutobackOn"() -> (w495:bool)
    n262 = local read "SBCOn"() -> (w762:bool)
    n263 = feedback #24(0.0) -> (w581:dbl)
    n264 = case shown="참" "DriveStart" {
      tunnel: [w1190 w1191] -> w579
      tunnel: w576 -> [w1190 _]
      tunnel: w581 -> [_ w1191]
      frame False {
      }
      frame True {
      }
    }
    n265 = feedback-in #24(w579) -> ()
    n266 = local read "AutobackOn"() -> (w449:bool)
    n267 = feedback #25(w831) -> (w832:dbl)
    n268 = case shown="거짓" w386 {
      tunnel: w639 -> [_ w1257]
      tunnel: [w1256 w1257] -> w830
      tunnel: w832 -> [w1256 _]
      frame False {
      }
      frame True {
      }
    }
    n269 = feedback-in #25(w830) -> ()
    n270 = feedback #26(w831) -> (w833:dbl)
    n271 = case shown="거짓" w386 {
      tunnel: [w1258 w1259] -> w829
      tunnel: w833 -> [w1258 _]
      tunnel: w639 -> [_ w1259]
      frame False {
      }
      frame True {
      }
    }
    n272 = feedback-in #26(w829) -> ()
    n273 = feedback #27(0.0) -> (w567:dbl)
    n274 = Subtract(x=w576, y=w579) -> (x-y=w573:dbl)
    n275 = formula code="float timer;\nif (nowV < v2 )\ntimer= -0.8*(nowV- v1)+t1;\nelse if (nowV >= v2)\ntimer= -0.667*(nowV- v2)+t2;\nelse \ntimer = 10.5;"("t1"=11.5 ("입력 변수"), "t2"=11.3 ("입력 변수"), "nowV"=w552, "v1"=2.1 ("입력 변수"), "v2"=2.35 ("입력 변수")) -> ("timer"=w547:dbl)
    "AutoTimer" <- w547
    n276 = feedback #28(0.0) -> (w998:dbl)
    n277 = formula code="if (u >165)\ny=165;\nelse if (u <-165)\ny=-165;\nelse\ny=u;"("u"=w838) -> ("y"=w825:dbl)
    n278 = Select(t="V_target", s="VelRef_0(off)", f=0.0) -> (s? t:f=w590:dbl)
    n279 = feedback #29(w831) -> (w834:dbl)
    n280 = case shown="거짓" w386 {
      tunnel: w639 -> [_ w1261]
      tunnel: [w1260 w1261] -> w828
      tunnel: w834 -> [w1260 _]
      frame False {
      }
      frame True {
      }
    }
    n281 = feedback-in #29(w828) -> ()
    n282 = feedback #30(0.0) -> (w393:dbl)
    "sum_y" <- w393
    n283 = Add(x=w523, y=w393) -> (x+y=w389:dbl)
    n284 = Select(t=0.0, s=w386, f=w389) -> (s? t:f=w388:dbl)
    n285 = feedback-in #30(w388) -> ()
    n286 = feedback #31(0.0) -> (w394:dbl)
    "DeltaX" <- w394
    "sum_x" <- w394
    n287 = Add(x=w526, y=w394) -> (x+y=w392:dbl)
    n288 = Select(t=0.0, s=w386, f=w392) -> (s? t:f=w391:dbl)
    n289 = feedback-in #31(w391) -> ()
    n290 = Select(t="Ang_ref\n1v=10deg", s="AngRef_0(off)", f=0.0) -> (s? t:f=w632:dbl)
    n291 = local read "AutobackVel"() -> (w503:dbl)
    n292 = Greater?(x=w573, y=w547) -> (0:w574:bool)
    n293 = Select(t=w552, s=w574, f=0.0) -> (s? t:f=w507:dbl)
    n294 = Compound Arithmetic op=ADD(w832, w833, w834) -> (w835:dbl)
    n295 = local read "AutobackOn"() -> (w508:bool)
    n296 = formula code="if ( 180 < u && y <=360)\ny = u-360;\nelse\ny = u;"("u"=w639) -> ("y"=w638:dbl)
    "NowAng" <- w638
    n297 = local read "Kt_rot"() -> (w1008:dbl)
    n298 = local read "SBCAutoback"() -> (w403:dbl)
    n299 = Divide(x=w835, y=3.0) -> (x/y=w827:dbl)
    n300 = local read "SBCvariable"() -> (w532:dbl)
    n301 = formula code="float phi_cmd,phi;\nphi=now_phi+ref_phi;\nif ( 180 < phi && phi <=360)\nphi_cmd = phi-360;\nelse\nphi_cmd = phi;"("ref_phi"=w825, "now_phi"=w827) -> ("phi_cmd"=w637:dbl)
    n302 = local read "Time"() -> (w793:i32)
    n303 = Select(t=w503, s=w449, f=w507) -> (s? t:f=w506:dbl)
    n304 = Select(t=w506, s="SBCOn", f=w590) -> (s? t:f=w651:dbl)
    "VelRef" <- w651
    n305 = Bundle("y0"=w922, "y0"=w921, "y0"=w919, w928, w927, w926, "MinW"=w924, "f"=w651) -> (→"Wheel_Vel":T14)  [unwired: 1 in]
    n306 = Divide(x=w793, y=1000) -> (x/y=w359:dbl)
    n307 = Equal?(x=w532, y=4.0) -> (x = y?=w360:bool)
    n308 = case shown="참" w360 {
      tunnel: [w1166 w1167] -> w362
      tunnel: w358 -> [_ w1167]
      tunnel: w359 -> [w1166 _]
      frame False {
      }
      frame True {
      }
    }
    n309 = feedback-in #21(w362) -> ()
    n310 = Subtract(x=w359, y=w362) -> (x-y=w361:dbl)
    n311 = Greater?(x=w361, y=0.0) -> (0:w366:bool)
    n312 = Less?(x=w361, y=1.0) -> (x < y?=w367:bool)
    n313 = And(x=w366, y=w367) -> (x .and. y?=w357:bool)
    n314 = Select(t=w355, s=w357, f=w354) -> (s? t:f=w353:dbl)
    n315 = Select(t=w353, s=w762, f=w632) -> (s? t:f=w518:dbl)
    n316 = local read "sum_y"() -> (w499:dbl)
    n317 = Multiply(x="PD_cut_rot", y=6.283185307179586) -> (x*y=w1022:dbl)
    n318 = local read "Vel_Robot"() -> (w453:dbl)
    n319 = local read "SBCdata3"() -> (w789:dbl)
    n320 = local read "SBCdata1"() -> (w791:dbl)
    n321 = local read "SBCdata2"() -> (w790:dbl)
    n322 = feedback #32(0.0) -> (w1025:dbl)
    n323 = Divide(x="J_FF_rot", y=w1008) -> (x/y=w1034:dbl)
    n324 = feedback #33(0.0) -> (w605:dbl)
    n325 = Equal?(x=w403, y=13.0) -> (x = y?=w509:bool)
    "AutobackOn" <- w509
    n326 = Reciprocal(x=w1022) -> (1/x=w1023:dbl)
    n327 = Select(t=w359, s=w360, f=0.0) -> (s? t:f=w541:dbl)
    n328 = local read "Pmod_YR"() -> (w1000:dbl)
    n329 = feedback #34(0.0) -> (w731:dbl)
    n330 = Multiply(x="FF_cut", y=6.283185307179586) -> (x*y=w1012:dbl)
    n331 = Bundle("f"=w651, "Vel_Robot"=w453) -> (→"Velocity":cluster{"f":dbl, "Vel_Robot":dbl})  [unwired: 1 in]
    n332 = local read "sum_x"() -> (w434:dbl)
    n333 = Greater?(x=w359, y=1.0) -> (0:w750:bool)
    n334 = Less?(x=w359, y=1.03) -> (x < y?=w749:bool)
    n335 = feedback #35(0.0 ("gy_z[]")) -> (w1017:dbl)
    n336 = Multiply(x="TxHz", y=6.283185307179586) -> (x*y=w540:dbl)
    n337 = Reciprocal(x=w1012) -> (1/x=w1014:dbl)
    n338 = And(x=w750, y=w749) -> (x .and. y?=w748:bool)
    n339 = Less?(x=w499, y="yStop") -> (x < y?=w494:bool)
    n340 = feedback #36(0.0 ("Vel_Robot")) -> (w451:dbl)
    n341 = case shown="참" w449 {
      tunnel: [w1171 w1172] -> w452
      tunnel: w453 -> [w1171 _]
      tunnel: w451 -> [_ w1172]
      frame False {
      }
      frame True {
      }
    }
    "NowVel13" <- w452
    n342 = feedback-in #36(w452) -> ()
    n343 = Multiply(x=w540, y=w541) -> (x*y=w542:dbl)
    n344 = Subtract(x=w651, y=w453) -> (x-y=w784:dbl)
    n345 = feedback #37(0.0) -> (w521:dbl)
    n346 = case shown="참" w509 {
      tunnel: w521 -> [_ w1186]
      tunnel: w359 -> [w1185 _]
      tunnel: [w1185 w1186] -> w520
      frame False {
      }
      frame True {
      }
    }
    n347 = feedback-in #37(w520) -> ()
    n348 = formula code="if (x > xu)\nphi=30;\nelse if (x < xd)\nphi=-30;\nelse \nphi=0;"("x"=w434, "xu"="upperx", "xd"="downx") -> ("phi"=w433:dbl)
    n349 = Sine(x=w542) -> (sin(x)=w535:dbl)
    "SinTx" <- w535
    n350 = feedback #38(0.0) -> (w477:dbl)
    n351 = local read "sum_y"() -> (w505:dbl)
    n352 = case shown="7" w397 {
      tunnel: w791 -> [w1219 w1231 w1238 _ _ _]
      tunnel: w790 -> [w1218 w1230 w1237 _ _ _]
      tunnel: w789 -> [w1217 w1229 w1236 _ _ _]
      tunnel: [FALSE ("SetSteer2Ori(On)") FALSE ("SetSteer2Ori(On)") FALSE ("SetSteer2Ori(On)") FALSE ("SetSteer2Ori(On)") FALSE ("SetSteer2Ori(On)") TRUE ("SetSteer2Ori(On)")] -> w686
      tunnel: [w1221 TRUE ("SetSteer2Ori(On)") w1234 w1241 w1246 FALSE ("SetSteer2Ori(On)")] -> w602
      tunnel: [w1221 TRUE ("SetSteer2Ori(On)") w1234 w1241 w1246 w1252] -> w560
      frame 2 {
        w1221 = FALSE ("SetSteer2Ori(On)")
        w1223 = 0.0 ("Steer_ang_ref[NoScale]")
        w1222 = FALSE ("DOBOnSBC")
        n353 = local write "DriveStart"(w1222) -> ()
        n354 = local write "Steer_ang_ref[NoScale]"(w1223) -> ()
        n355 = local write "Vel_cmd"(w1223) -> ()
        n356 = local write "Yawangle*"(w1223) -> ()
        n357 = local write "DOBOnSBC"(w1222) -> ()
        n358 = local write "SBC2mode"(FALSE ("SBCSteerEnable")) -> ()
        "SBCDriveEnable" <- FALSE ("SBCDriveEnable")
        "Steer1NowAbs 2" <- w1219
        "Steer2NowAbs" <- w1218
        "Steer3NowAbs" <- w1217
      }
      frame 3 {
        n359 = local write "SBCDriveEnable"(TRUE ("SBCDriveEnable")) -> ()
        "Steer_ang_ref[NoScale]" <- w1230
        "Yawangle*" <- w1229
        "Vel_cmd" <- w1231
        "SBC2mode" <- TRUE ("SBCSteerEnable")
      }
      frame 4, Default {
        w1234 = FALSE ("SetSteer2Ori(On)")
        n360 = local write "Vel_cmd"(w1238) -> ()
        n361 = local write "Steer_ang_ref[NoScale]"(w1237) -> ()
        n362 = local write "Yawangle*"(w1236) -> ()
        n363 = local write "SBCDriveEnable"(TRUE ("SBCDriveEnable")) -> ()
        n364 = local write "SBC2mode"(TRUE ("SBCSteerEnable")) -> ()
      }
      frame 5 {
        w1241 = FALSE ("SetSteer2Ori(On)")
        w1242 = FALSE ("SBCDriveEnable")
        n365 = local write "SBCDriveEnable"(w1242) -> ()
        n366 = local write "DOBOnSBC"(FALSE ("DOBOnSBC")) -> ()
        n367 = local write "SBC2mode"(TRUE ("SBCSteerEnable")) -> ()
        n368 = local write "DriveStart"(w1242) -> ()
      }
      frame 6 {
        w1246 = FALSE ("SetSteer2Ori(On)")
        n369 = local write "DriveStart"(TRUE ("SBCDrivingStart")) -> ()
        n370 = local write "SBC2mode"(TRUE ("SBCSteerEnable")) -> ()
        "DOBOnSBC" <- TRUE ("DOBOnSBC")
      }
      frame 7 {
        w1252 = FALSE ("SBCDrivingStart")
        w1250 = 0.0 ("Steer_ang_ref[NoScale]")
        n371 = local write "Vel_cmd"(w1250) -> ()
        n372 = local write "Steer_ang_ref[NoScale]"(w1250) -> ()
        n373 = local write "SBCAutoback"(w1250) -> ()
        n374 = local write "Yawangle*"(w1250) -> ()
        n375 = local write "DriveStart"(w1252) -> ()
        n376 = local write "SBCDriveEnable"(w1252) -> ()
        n377 = local write "DOBOnSBC"(FALSE ("DOBOnSBC")) -> ()
        n378 = local write "SBC2mode"(TRUE ("SBCSteerEnable")) -> ()
      }
    }
    n379 = case shown="참" w560 {
      tunnel: [w1188 w1189] -> w563
      tunnel: w567 -> [_ w1189]
      tunnel: w359 -> [w1188 _]
      frame False {
      }
      frame True {
      }
    }
    n380 = feedback-in #27(w563) -> ()
    n381 = Subtract(x=w359, y=w563) -> (x-y=w562:dbl)
    n382 = Greater?(x=w562, y=0.0) -> (0:w568:bool)
    n383 = Less?(x=w562, y=1.0) -> (x < y?=w569:bool)
    n384 = And(x=w568, y=w569) -> (x .and. y?=→"SBCAngReset":bool)
    n385 = case shown="참" w602 {
      tunnel: [w1204 w1205] -> w609
      tunnel: w605 -> [_ w1205]
      tunnel: w359 -> [w1204 _]
      frame False {
      }
      frame True {
      }
    }
    n386 = feedback-in #33(w609) -> ()
    n387 = Subtract(x=w359, y=w609) -> (x-y=w610:dbl)
    n388 = Greater?(x=w610, y=0.0) -> (0:w604:bool)
    n389 = Less?(x=w610, y=1.0) -> (x < y?=w603:bool)
    n390 = And(x=w604, y=w603) -> (x .and. y?=w555:bool)
    n391 = feedback #39(0.0) -> (w986:dbl)
    n392 = feedback-in #39(w637) -> ()
    n393 = feedback #40(FALSE) -> (w709:bool)
    n394 = case shown="참" w709 {
      tunnel: [w1212 w1213] -> w726
      tunnel: w359 -> [w1212 _]
      tunnel: w731 -> [_ w1213]
      frame False {
      }
      frame True {
      }
    }
    n395 = feedback-in #34(w726) -> ()
    n396 = Subtract(x=w359, y=w726) -> (x-y=w725:dbl)
    n397 = Greater?(x=w725, y=0.0) -> (0:w732:bool)
    n398 = Less?(x=w725, y=0.003) -> (x < y?=w733:bool)
    n399 = And(x=w732, y=w733) -> (x .and. y?=w728:bool)
    n400 = Greater?(x=w535, y=0.0) -> (0:w536:bool)
    n401 = Subtract(x=w359, y=w520) -> (x-y=w401:dbl)
    "Time_autoback" <- w401
    n402 = Greater?(x=w401, y=8.0) -> (0:w431:bool)
    n403 = Less?(x=w401, y=13.0) -> (x < y?=w432:bool)
    n404 = Greater?(x=w401, y=1.0) -> (0:w419:bool)
    n405 = Less Or Equal?(x=w401, y=3.0) -> (x <= y?=w418:bool)
    n406 = Greater?(x=w401, y=8.0) -> (0:w400:bool)
    n407 = Compound Arithmetic op=AND ("복합 연산")(w400, w495, w494) -> (→"CompleteAutoback":bool)
    n408 = And(x=w431, y=w432) -> (x .and. y?=w426:bool)
    n409 = And(x=w419, y=w418) -> (x .and. y?=w424:bool)
    n410 = Boolean To (0,1)(Boolean=w426) -> (0, 1=w427:i16)
    n411 = Boolean To (0,1)(Boolean=w424) -> (0, 1=w423:i16)
    n412 = Multiply(x=w427, y=i16 10) -> (x*y=w425:i16)
    n413 = Multiply(x=w423, y=i16 5) -> (x*y=w417:i16)
    n414 = Greater?(x=w401, y=3.0) -> (0:w445:bool)
    n415 = Greater?(x=w401, y=0.0) -> (0:w515:bool)
    n416 = Less?(x=w401, y=8.0) -> (x < y?=w444:bool)
    n417 = Less?(x=w401, y=1.0) -> (x < y?=w513:bool)
    n418 = And(x=w445, y=w444) -> (x .and. y?=w437:bool)
    n419 = Compound Arithmetic op=AND ("복합 연산")(w515, w513, w509) -> (w441:bool)
    n420 = Boolean To (0,1)(Boolean=w437) -> (0, 1=w438:i16)
    n421 = Boolean To (0,1)(Boolean=w441) -> (0, 1=w443:i16)
    n422 = Multiply(x=w438, y=i16 8) -> (x*y=w436:i16)
    n423 = Multiply(x=w443, y=i16 2) -> (x*y=w440:i16)
    n424 = Compound Arithmetic op=ADD(w417, w440, w436, w425) -> (w385:i16)
    "AutobackCmd" <- w385
    n425 = case shown="2" w385 {
      tunnel: [-0.5 ("NowVel13") 0.0 ("NowVel13") -2.3 ("NowVel13") w1184] -> w407
      frame 8 {
      }
      frame 5 {
      }
      frame 10, Default {
      }
      frame 2 {
        n426 = local read "NowVel13"() -> (w1184:dbl)
      }
    }
    n427 = case shown="2" w385 {
      tunnel: [40.0 ("t") 40.0 ("phi") 0.0 ("t") w1176 0.0 ("phi")] -> w435
      tunnel: w433 -> [_ _ _ w1176 _]
      frame 2 {
      }
      frame 5 {
      }
      frame 0 {
      }
      frame 8 {
      }
      frame 10, Default {
      }
    }
    n428 = feedback-in #38(w435) -> ()
    n429 = local read "Yawangle"() -> (w622:dbl)
    n430 = feedback #41(0.0) -> (w775:dbl)
    n431 = case shown="참" w728 {
      tunnel: [w1214 w1215] -> w773
      tunnel: w359 -> [_ w1215]
      tunnel: w775 -> [w1214 _]
      frame False {
      }
      frame True {
      }
    }
    n432 = feedback-in #41(w773) -> ()
    n433 = Select(t=0.0, s=w494, f=-0.7 ("t")) -> (s? t:f=w498:dbl)
    n434 = Divide(x=w784, y=0.125) -> (x/y=w782:dbl)
    n435 = Greater?(x=w840, y=42000) -> (0:w843:bool)
    n436 = Unbundle(w896) -> ("y0"=w866:dbl, "y0"=w865:dbl, "y0"=w864:dbl)
    n437 = Greater?(x=w840, y=32000) -> (0:w845:bool)
    n438 = Multiply(x=0.5 ("PhiAngCUT 2"), y=6.283185307179586) -> (x*y=w473:dbl)
    n439 = Greater?(x=w840, y=52000) -> (0:w852:bool)
    n440 = local read "sum_x"() -> (w412:dbl)
    n441 = Multiply(x="PhiAngCUT", y=6.283185307179586) -> (x*y=w982:dbl)
    n442 = Greater?(x=w401, y=0.0) -> (0:w414:bool)
    n443 = Less Or Equal?(x=w401, y=3.0) -> (x <= y?=w413:bool)
    n444 = Reciprocal(x=w473) -> (1/x=w471:dbl)
    n445 = Subtract(x=w359, y=w773) -> (x-y=w714:dbl)
    n446 = Divide(x="B_FF_rot 2", y=w1008) -> (x/y=w1035:dbl)
    n447 = Reciprocal(x=w982) -> (1/x=w980:dbl)
    n448 = And(x=w414, y=w413) -> (x .and. y?=w409:bool)
    n449 = Less?(x=w505, y=5.0) -> (x < y?=w501:bool)
    n450 = Greater?(x=w412, y="LImitX") -> (0:w410:bool)
    n451 = Subtract(x=w782, y=w866) -> (x-y=w649:dbl)
    n452 = Subtract(x=w782, y=w865) -> (x-y=w647:dbl)
    n453 = Subtract(x=w782, y=w864) -> (x-y=w646:dbl)
    n454 = Boolean To (0,1)(Boolean=w536) -> (0, 1=w546:i16)
    n455 = And(x=w410, y=w409) -> (x .and. y?=w405:bool)
    n456 = Select(t=0.0, s=w405, f=w407) -> (s? t:f=w406:dbl)
    n457 = Select(t=w498, s=w501, f=w406) -> (s? t:f=→"AutobackVel":dbl)
    n458 = feedback #42(0.0 ("gy_z[]")) -> (w1015:dbl)
    n459 = feedback #43(0.0) -> (w1096:dbl)
    n460 = feedback-in #43(w1000) -> ()
    n461 = Greater?(x=w714, y=1.0) -> (0:w757:bool)
    n462 = Less?(x=w714, y=1.03) -> (x < y?=w756:bool)
    n463 = Multiply(x=w546, y=i16 1) -> (x*y=w544:i16)
    n464 = feedback #44() -> (w1030:dbl)  [unwired: 1 in]
    n465 = And(x=w757, y=w756) -> (x .and. y?=w553:bool)
    n466 = Or(x=w553, y=w555) -> (x .or. y?=→"SBCEncReset":bool)
    n467 = Or(x=w553, y=w748) -> (x .or. y?=w673:bool)
    "AskSBC4ABS" <- w673
    n468 = Boolean To (0,1)(Boolean=w673) -> (0, 1=w778:i16)
    n469 = Multiply(x=w778, y=i16 2) -> (x*y=w663:i16)
    n470 = local read "Steer2NowAbs"() -> (w742:dbl)
    n471 = local read "Steer1NowAbs 2"() -> (w739:dbl)
    n472 = local read "Steer3NowAbs"() -> (w736:dbl)
    n473 = Divide(x="J_FF_R_wh", y="Kt_longi") -> (x/y=w885:dbl)
    n474 = feedback #45(w853) -> (w846:dbl)
    n475 = case shown="참" w843 {
      tunnel: w622 -> [w1274 _]
      tunnel: [w1274 w1275] -> w618
      tunnel: w846 -> [_ w1275]
      frame False {
      }
      frame True {
      }
    }
    n476 = feedback-in #45(w618) -> ()
    n477 = feedback #46(w853) -> (w850:dbl)
    n478 = case shown="참" w852 {
      tunnel: w622 -> [w1262 _]
      tunnel: [w1262 w1263] -> w619
      tunnel: w850 -> [_ w1263]
      frame False {
      }
      frame True {
      }
    }
    n479 = feedback-in #46(w619) -> ()
    n480 = Divide(x="J_FF_R_wh", y="Kt_longi") -> (x/y=w888:dbl)
    n481 = Boolean To (0,1)(Boolean=w360) -> (0, 1=w594:i16)
    n482 = Divide(x="J_FF_R_wh", y="Kt_longi") -> (x/y=w904:dbl)
    n483 = Multiply(x=w646, y="Kp_wheelomega_Cont") -> (x*y=w643:dbl)
    n484 = Multiply(x=w647, y="Kp_wheelomega_Cont") -> (x*y=w644:dbl)
    n485 = feedback #47(0.0 ("gy_ratelimit")) -> (w1079:dbl)
    n486 = Greater?(x=w714, y=1.2) -> (0:w711:bool)
    n487 = Less?(x=w714, y=5.0) -> (x < y?=w710:bool)
    n488 = Multiply(x=w649, y="Kp_wheelomega_Cont") -> (x*y=w648:dbl)
    n489 = Multiply(x=w594, y=i16 4) -> (x*y=w543:i16)
    n490 = Bundle(w535, w544, w543) -> ()  [unwired: 1 in, 1 out]
    n491 = Multiply(x="right wheel FF_cut 2", y=6.283185307179586) -> (x*y=w878:dbl)
    n492 = Greater?(x=w359, y=1.1) -> (0:w712:bool)
    n493 = Less?(x=w359, y=5.1) -> (x < y?=w772:bool)
    n494 = Multiply(x=0.05 ("gy_offset_remover cutoff"), y=6.283185307179586) -> (x*y=w1101:dbl)
    n495 = Multiply(x="right wheel FF_cut 2", y=6.283185307179586) -> (x*y=w895:dbl)
    n496 = feedback #48(0.0 ("gy_z[]")) -> (w882:dbl)
    n497 = feedback-in #48(w782) -> ()
    n498 = Multiply(x="right wheel FF_cut 2", y=6.283185307179586) -> (x*y=w897:dbl)
    n499 = local read "SetSteer2Ori(On)"() -> (w788:bool)
    n500 = feedback #49(w853) -> (w847:dbl)
    n501 = case shown="참" w845 {
      tunnel: w622 -> [w1272 _]
      tunnel: [w1272 w1273] -> w617
      tunnel: w847 -> [_ w1273]
      frame False {
      }
      frame True {
      }
    }
    n502 = feedback-in #49(w617) -> ()
    n503 = feedback #50(0.0) -> (w1072:dbl)
    n504 = feedback #51(0.0 ("gy_z[]")) -> (w891:dbl)
    n505 = feedback-in #51(w782) -> ()
    n506 = feedback #52(0.0 ("gy_z[]")) -> (w901:dbl)
    n507 = feedback-in #52(w782) -> ()
    n508 = Compound Arithmetic op=AND ("복합 연산")(w711, w710) -> (w713:bool)
    n509 = feedback #53(0.0) -> (w476:dbl)
    n510 = formula code="float F,A,B,C,y0;\nF=2*tau+T;\nA=(2*a+b*T)/F;\nB=(b*T-2*a)/F;\nC=(2*tau-T)/F;\ny0=A*u0+B*u1+C*y1;"("tau"=w471, "u0"=w435, "u1"=w477, "y1"=w476, "T"=0.001 ("input variable"), "a"=0.0 ("input variable"), "b"=1.0 ("input variable")) -> ("y0"=w468:dbl)
    n511 = Select(t=w468, s=w508, f=w518) -> (s? t:f=w517:dbl)
    "RearSteerCmd" <- w517
    n512 = Negate(x=w517) -> (-x=w670:dbl)
    n513 = feedback-in #53(w468) -> ()
    n514 = Reciprocal(x=w878) -> (1/x=w880:dbl)
    n515 = Reciprocal(x=w895) -> (1/x=w893:dbl)
    n516 = Reciprocal(x=w897) -> (1/x=w899:dbl)
    n517 = And(x=w712, y=w772) -> (x .and. y?=w755:bool)
    n518 = Reciprocal(x=w1101) -> (1/x=w1093:dbl)
    n519 = feedback #54(0.0) -> (w985:dbl)
    n520 = formula code="float F,A,B,C,y0;\nF=2*tau+T;\nA=(2*a+b*T)/F;\nB=(b*T-2*a)/F;\nC=(2*tau-T)/F;\ny0=A*u0+B*u1+C*y1;"("tau"=w980, "u0"=w637, "u1"=w986, "y1"=w985, "T"=0.001 ("input variable"), "a"=0.0 ("input variable"), "b"=1.0 ("input variable")) -> ("y0"=w977:dbl)
    "AngRer" <- w977
    n521 = Bundle(w977, "y"=w638, "Yawangle*"=w557) -> (→"Yaw angle":cluster{dbl, "y":dbl, "Yawangle*":dbl})  [unwired: 1 in]
    n522 = Subtract(x=w977, y=w638) -> (x-y=w636:dbl)
    n523 = formula code="if (u >3)\ny=3;\nelse if (u <-3)\ny=-3;\nelse\ny=u;"("u"=w636) -> ("y"=w635:dbl)
    n524 = feedback-in #22(w635) -> ()
    n525 = formula code="float F,A,B,C,ykd,ykp,y0;\nF=2*tau+T;\nA=(2*Kd_rot)/F;\nB=(-2*Kd_rot)/F;\nC=(2*tau-T)/F;\nykd=A*u0+B*u1+C*y1;\nykp=Kp_rot*u0;\ny0=ykp+ykd;"("tau"=w992, "u0"=w635, "u1"=w994, "y1"=w998, "T"=0.001 ("input variable"), "Kp_rot"="Kp_rot 3", "Kd_rot"="Kd_rot 4") -> ("y0"=w971:dbl)
    n526 = feedback-in #28(w971) -> ()
    n527 = feedback-in #54(w977) -> ()
    n528 = Subtract(x="Steer2OriAbs 2", y=w742) -> (x-y=w741:dbl)
    n529 = Subtract(x="Steer1OriAbs", y=w739) -> (x-y=w738:dbl)
    n530 = Subtract(x="Steer3OriAbs 3", y=w736) -> (x-y=w735:dbl)
    n531 = Multiply(x=w738, y="90/10\nRealAng") -> (x*y=w737:dbl)
    n532 = local read "SBC2mode"() -> (w534:bool)
    n533 = Multiply(x=w735, y="90/10\nRealAng") -> (x*y=w734:dbl)
    n534 = Less?(x=w359, y=22.0) -> (x < y?=w707:bool)
    n535 = Multiply(x="0.1V/deg", y=w670) -> (x*y=w668:dbl)
    n536 = Multiply(x="90/10\nRealAng", y=w741) -> (x*y=w740:dbl)
    n537 = Greater?(x=w714, y=5.0) -> (0:w691:bool)
    n538 = Less?(x=w714, y=5.2) -> (x < y?=w690:bool)
    n539 = Subtract(x=w618, y=w617) -> (x-y=w854:dbl)
    n540 = Subtract(x=w619, y=w618) -> (x-y=w855:dbl)
    n541 = Multiply(x="ratelimit cut", y=6.283185307179586) -> (x*y=w1075:dbl)
    n542 = Multiply(x=w737, y="0.1V/deg") -> (x*y=w671:dbl)
    n543 = Multiply(x=w740, y="0.1V/deg") -> (x*y=w723:dbl)
    n544 = local read "Vel_Robot"() -> (w818:dbl)
    n545 = feedback #55(0.0) -> (w1100:dbl)
    n546 = formula code="float F,A,B,C,y0;\nF=2*tau+T;\nA=(2*a+b*T)/F;\nB=(b*T-2*a)/F;\nC=(2*tau-T)/F;\ny0=A*u0+B*u1+C*y1;"("tau"=w1093, "u0"=w1000, "u1"=w1096, "y1"=w1100, "T"=0.001 ("input variable"), "a"=0.0 ("input variable"), "b"=1.0 ("input variable")) -> ("y0"=w1005:dbl)
    n547 = feedback-in #55(w1005) -> ()
    n548 = feedback #56(0.0) -> (w969:dbl)
    n549 = Reciprocal(x=w1075) -> (1/x=w1074:dbl)
    n550 = Add(x=w854, y=w855) -> (x+y=w856:dbl)
    n551 = local read "DOBOnSBC"() -> (w570:bool)
    n552 = Or(x=w570, y="YR*_zero(off)") -> (x .or. y?=w571:bool)
    n553 = Select(t=w971, s=w571, f=0.0) -> (s? t:f=w972:dbl)
    n554 = feedback-in #35(w972) -> ()
    n555 = formula code="float F,A,B,C,y0;\nF=2*tau+T;\nA=(2*a+b*T)/F;\nB=(b*T-2*a)/F;\nC=(2*tau-T)/F;\ny0=A*u0+B*u1+C*y1;"("tau"=w1014, "u0"=w972, "u1"=w1017, "y1"=w1015, "T"=0.001 ("input variable"), "a"=w1034, "b"=w1035) -> ("y0"=w975:dbl)
    n556 = feedback-in #42(w975) -> ()
    n557 = Tick Count (ms)() -> (millisecond timer value=w585:u32)
    n558 = Multiply(x=w734, y="0.1V/deg") -> (x*y=w722:dbl)
    n559 = local read "AskSBC4ABS"() -> (w776:bool)
    n560 = Absolute Value(x=w737) -> (abs(x)=w797:dbl)
    n561 = Select(t=w671, s=w788, f=w668) -> (s? t:f=w801:dbl)
    n562 = Divide(x="B_FF_R_wh", y="Kt_longi") -> (x/y=w886:dbl)
    n563 = Absolute Value(x=w818) -> (abs(x)=w820:dbl)
    n564 = Greater?(x=w820, y=0.05) -> (0:w769:bool)
    n565 = Divide(x=w856, y=2.0) -> (x/y=w858:dbl)
    n566 = Divide(x="B_FF_R_wh", y="Kt_longi") -> (x/y=w887:dbl)
    n567 = Divide(x="B_FF_R_wh", y="Kt_longi") -> (x/y=w905:dbl)
    n568 = Select(t=w723, s=w788, f=w668) -> (s? t:f=w799:dbl)
    n569 = Select(t=w722, s=w788, f=w668) -> (s? t:f=w798:dbl)
    n570 = feedback #57() -> (w584:u32)  [unwired: 1 in]
    n571 = feedback-in #57(w585) -> ()
    n572 = feedback #58(0.0) -> (w699:dbl)
    n573 = case shown="참" w686 {
      tunnel: [w1208 w1209] -> w704
      tunnel: w699 -> [_ w1209]
      tunnel: w359 -> [w1208 _]
      frame False {
      }
      frame True {
      }
    }
    n574 = feedback-in #58(w704) -> ()
    n575 = Greater?(x=w818, y=0.0) -> (0:w823:bool)
    n576 = Or(x="YRContDOB", y=w570) -> (x .or. y?=w765:bool)
    n577 = Absolute Value(x=w740) -> (abs(x)=w796:dbl)
    n578 = feedback #59(0.0) -> (w679:dbl)
    n579 = feedback #60(0.0 ("gy_z[]")) -> (w881:dbl)
    n580 = formula code="float F,A,B,C,y0;\nF=2*tau+T;\nA=(2*a+b*T)/F;\nB=(b*T-2*a)/F;\nC=(2*tau-T)/F;\ny0=A*u0+B*u1+C*y1;"("tau"=w880, "u0"=w782, "u1"=w882, "y1"=w881, "T"=0.001 ("input variable"), "a"=w885, "b"=w886) -> ("y0"=w874:dbl)
    n581 = feedback-in #60(w874) -> ()
    n582 = Subtract(x=w359, y=w704) -> (x-y=w705:dbl)
    n583 = feedback #61(0.0) -> (w1077:dbl)
    n584 = feedback #62(0.0 ("gy_z[]")) -> (w892:dbl)
    n585 = formula code="float F,A,B,C,y0;\nF=2*tau+T;\nA=(2*a+b*T)/F;\nB=(b*T-2*a)/F;\nC=(2*tau-T)/F;\ny0=A*u0+B*u1+C*y1;"("tau"=w893, "u0"=w782, "u1"=w891, "y1"=w892, "T"=0.001 ("input variable"), "a"=w888, "b"=w887) -> ("y0"=w872:dbl)
    n586 = feedback-in #62(w872) -> ()
    n587 = feedback #63(0.0 ("gy_z[]")) -> (w900:dbl)
    n588 = formula code="float F,A,B,C,y0;\nF=2*tau+T;\nA=(2*a+b*T)/F;\nB=(b*T-2*a)/F;\nC=(2*tau-T)/F;\ny0=A*u0+B*u1+C*y1;"("tau"=w899, "u0"=w782, "u1"=w901, "y1"=w900, "T"=0.001 ("input variable"), "a"=w904, "b"=w905) -> ("y0"=w875:dbl)
    n589 = Add(x=w648, y=w875) -> (x+y=w867:dbl)
    n590 = feedback-in #63(w875) -> ()
    n591 = Absolute Value(x=w734) -> (abs(x)=w795:dbl)
    n592 = Not(x=w776) -> (.not. x?=w770:bool)
    n593 = Add(x=w644, y=w872) -> (x+y=w869:dbl)
    n594 = Less?(x=w797, y="AbsErrorCrit") -> (x < y?=w720:bool)
    n595 = Less?(x=w796, y="AbsErrorCrit") -> (x < y?=w719:bool)
    n596 = Greater?(x=w705, y=0.0) -> (0:w698:bool)
    n597 = Subtract(x=w585, y=w584) -> (x-y=→"loopTime" →"Timing":u32)
    n598 = Add(x=w874, y=w643) -> (x+y=w871:dbl)
    n599 = Less?(x=w705, y=0.003) -> (x < y?=w697:bool)
    n600 = Less?(x=w795, y="AbsErrorCrit") -> (x < y?=w718:bool)
    n601 = Greater?(x=w840, y=44000) -> (0:w1089:bool)
    n602 = Greater?(x=w840, y=32000) -> (0:w1094:bool)
    n603 = Select(t=w769, s=w765, f=FALSE) -> (s? t:f=w768:bool)
    n604 = Select(t=w975, s=w768, f=0.0) -> (s? t:f=w974:dbl)
    n605 = And(x=w698, y=w697) -> (x .and. y?=w702:bool)
    n606 = Greater?(x=w840, y=56000) -> (0:w1088:bool)
    n607 = Compound Arithmetic op=OR ("복합 연산")(w713, w755, "SetSteer") -> (w759:bool)
    "SetSteer2Ori(On)" <- w759
    n608 = Or(x=w534, y=w759) -> (x .or. y?=→"SBCSteerEnable":bool)
    n609 = Compound Arithmetic op=AND ("복합 연산")(w770, w720, w719, w718) -> (w672:bool)
    "CompliteABS" <- w672
    n610 = case shown="참" w672 {
      tunnel: [w1206 w1207] -> w675
      tunnel: w679 -> [_ w1207]
      tunnel: w359 -> [w1206 _]
      frame False {
      }
      frame True {
      }
    }
    n611 = feedback-in #59(w675) -> ()
    n612 = Subtract(x=w359, y=w675) -> (x-y=w674:dbl)
    n613 = Greater?(x=w674, y=1.0) -> (0:w680:bool)
    n614 = Less?(x=w674, y=1.03) -> (x < y?=w681:bool)
    n615 = feedback #64(0.0) -> (w1053:dbl)
    n616 = feedback-in #64(w969) -> ()
    n617 = Compound Arithmetic op=AND ("복합 연산")(w720, w719, w718) -> (w716:bool)
    n618 = Not(x=w716) -> (.not. x?=w689:bool)
    n619 = Compound Arithmetic op=AND ("복합 연산")(w691, w690, w689, w707) -> (w685:bool)
    n620 = feedback #65(0.0 ("gy_z[]")) -> (w1050:dbl)
    n621 = Greater?(x=w840, y=53000) -> (0:w849:bool)
    n622 = And(x=w680, y=w681) -> (x .and. y?=w370:bool)
    n623 = Boolean To (0,1)(Boolean=w370) -> (0, 1=w664:i16)
    n624 = Multiply(x=w664, y=i16 8) -> (x*y=w662:i16)
    n625 = feedback #66(0.0) -> (w694:dbl)
    n626 = case shown="거짓" w702 {
      tunnel: [w1210 w1211] -> w696
      tunnel: w359 -> [_ w1211]
      tunnel: w694 -> [w1210 _]
      frame False {
      }
      frame True {
      }
    }
    n627 = feedback-in #66(w696) -> ()
    n628 = case shown="참" w849 {
      tunnel: [180 w1270] -> w621
      tunnel: w622 -> [_ w1266]
      tunnel: w840 -> [_ w1268]
      tunnel: w858 -> [_ w1265]
      frame False {
      }
      frame True {
        n629 = Divide(x=w1265, y=10000) -> (x/y=w1269:dbl)
        n630 = Multiply(x=w1269, y=w1268) -> (x*y=w1267:dbl)
        n631 = Subtract(x=w1266, y=w1267) -> (x-y=w1270:dbl)
        "bias per 0.5min" <- w1265
      }
    }
    n632 = Subtract(x=w359, y=w696) -> (x-y=w692:dbl)
    n633 = local read "CompleteAutoback"() -> (w484:bool)
    n634 = Divide(x="Jm_rot", y="Kt_rot") -> (x/y=w1048:dbl)
    n635 = Less?(x=w692, y=22.0) -> (x < y?=w688:bool)
    n636 = Compound Arithmetic op=AND ("복합 연산")(w691, w690, w689, w688) -> (w684:bool)
    n637 = Compound Arithmetic op=OR ("복합 연산")(w686, w685, w684) -> (w687:bool)
    n638 = feedback-in #40(w687) -> ()
    n639 = Multiply(x="DOB_FB_cut", y=6.283185307179586) -> (x*y=w1054:dbl)
    n640 = Reciprocal(x=w1054) -> (1/x=w1056:dbl)
    n641 = local read "Tqoff_autoback"() -> (w510:bool)
    n642 = feedback #67(w1085) -> (w1082:dbl)
    n643 = case shown="거짓" w1094 {
      tunnel: w1005 -> [w1280 _]
      tunnel: [w1280 w1281] -> w1092
      tunnel: w1082 -> [_ w1281]
      frame False {
      }
      frame True {
      }
    }
    n644 = feedback-in #67(w1092) -> ()
    n645 = feedback #68(w1085) -> (w1084:dbl)
    n646 = case shown="참" w1088 {
      tunnel: w1005 -> [w1276 _]
      tunnel: [w1276 w1277] -> w1086
      tunnel: w1084 -> [_ w1277]
      frame False {
      }
      frame True {
      }
    }
    n647 = feedback-in #68(w1086) -> ()
    n648 = feedback #69(w1085) -> (w1083:dbl)
    n649 = case shown="참" w1089 {
      tunnel: w1005 -> [w1278 _]
      tunnel: [w1278 w1279] -> w1087
      tunnel: w1083 -> [_ w1279]
      frame False {
      }
      frame True {
      }
    }
    n650 = feedback-in #69(w1087) -> ()
    n651 = Divide(x="Bm_rot", y="Kt_rot") -> (x/y=w1047:dbl)
    n652 = feedback #70(0.0 ("Steer_ang_ref[NoScale]")) -> (w807:dbl)
    n653 = feedback-in #70(w801) -> ()
    n654 = feedback #71(0.0 ("Steer_ang_ref[NoScale]")) -> (w914:dbl)
    n655 = feedback-in #71(w798) -> ()
    n656 = feedback #72(0.0 ("Steer_ang_ref[NoScale]")) -> (w810:dbl)
    n657 = feedback-in #72(w799) -> ()
    n658 = Multiply(x="Steer_ang*_cut 2", y=6.283185307179586) -> (x*y=w908:dbl)
    n659 = Reciprocal(x=w908) -> (1/x=w800:dbl)
    n660 = feedback #73(0.0) -> (w487:dbl)
    n661 = case shown="참" w484 {
      tunnel: [w1179 w1180] -> w491
      tunnel: w487 -> [_ w1180]
      tunnel: w359 -> [w1179 _]
      frame False {
      }
      frame True {
      }
    }
    n662 = feedback-in #73(w491) -> ()
    n663 = local read "AskSBC"() -> (w601:i16)
    "send2SBC1" <- w601
    n664 = case shown="13" w601 {
      tunnel: [0.0 ("NowAng") 0.0 ("NowAng") 0.0 ("NowAng") 0.0 ("NowAng")] -> w600
      tunnel: [w1193 w1197 w1199 w1203] -> w599
      tunnel: [w1194 w1196 w1200 w1202] -> w598
      frame 2 {
        n665 = local read "x_Rear"() -> (w1193:dbl)
        n666 = local read "Vel_Robot"() -> (w1194:dbl)
      }
      frame 9, Default {
        n667 = local read "x_Rear"() -> (w1197:dbl)
        n668 = local read "Vel_Robot"() -> (w1196:dbl)
      }
      frame 13 {
        n669 = local read "Vel_Robot"() -> (w1200:dbl)
        n670 = local read "x_Rear"() -> (w1199:dbl)
      }
      frame 8 {
        n671 = local read "Vel_Robot"() -> (w1202:dbl)
        n672 = local read "x_Rear"() -> (w1203:dbl)
      }
    }
    "send2SBC 2" <- w600
    "send2SBC 3" <- w599
    "send2SBC 4" <- w598
    n673 = Compound Arithmetic op=ADD(w1084, w1083, w1082) -> (w1081:dbl)
    n674 = And(x="TqOn(On)", y=w510) -> (x .and. y?=w511:bool)
    n675 = Subtract(x=w359, y=w491) -> (x-y=w492:dbl)
    n676 = feedback #74(0.0) -> (w1052:dbl)
    n677 = formula code="float F,A,B,C,y0;\nF=2*tau+T;\nA=(2*a+b*T)/F;\nB=(b*T-2*a)/F;\nC=(2*tau-T)/F;\ny0=A*u0+B*u1+C*y1;"("tau"=w1056, "u0"=w969, "u1"=w1053, "y1"=w1052, "T"=w1051, "a"=0.0 ("input variable"), "b"=1.0 ("input variable")) -> ("y0"=w1040:dbl)
    n678 = feedback-in #74(w1040) -> ()
    n679 = feedback #75(0.0) -> (w1049:dbl)
    n680 = formula code="if (ang > 360)\nang1=ang-360;\nelse\nang1=ang;"("ang"=w621) -> ("ang1"=→"YawAngFB":dbl)
    n681 = Greater?(x=w492, y=1.0) -> (0:w486:bool)
    n682 = Less?(x=w492, y=1.03) -> (x < y?=w485:bool)
    n683 = Divide(x=w1081, y=3.0) -> (x/y=w1004:dbl)
    n684 = Subtract(x=w1000, y=w1004) -> (x-y=w1003:dbl)
    n685 = formula code="float rate;\nrate=gy-gy_r1;\nif (rate > limit)\ngy_ratelimit=gy_r1+limit;\nelse if (rate < -limit)\ngy_ratelimit=gy_r1+(-limit);\nelse\ngy_ratelimit=gy;"("gy"=w1003, "gy_r1"=w1079, "limit"="yaw_ratelimit") -> ("gy_ratelimit"=w1064:dbl)
    n686 = feedback-in #47(w1064) -> ()
    n687 = feedback-in #50(w1064) -> ()
    n688 = formula code="float F,A,B,C,y0;\nF=2*tau+T;\nA=(2*a+b*T)/F;\nB=(b*T-2*a)/F;\nC=(2*tau-T)/F;\ny0=A*u0+B*u1+C*y1;"("tau"=w1074, "u0"=w1064, "u1"=w1072, "y1"=w1077, "T"=0.001 ("input variable"), "a"=0.0 ("input variable"), "b"=1.0 ("input variable")) -> ("y0"=w1067:dbl)
    n689 = feedback-in #61(w1067) -> ()
    n690 = formula code="float band_ratelim;\n\nif (gy_ratelim < gy_band && gy_ratelim > -gy_band)\nband_ratelim=0;\nelse\nband_ratelim=gy_ratelim;"("gy_ratelim"=w1067, "gy_band"="ratelimit band") -> ("band_ratelim"=w1002:dbl)
    n691 = And(x=w486, y=w485) -> (x .and. y?=w481:bool)
    n692 = Compound Arithmetic op=OR ("복합 연산")(w673, w370, w536, w481) -> (w761:bool)
    n693 = local write "SendDataOn"(w761) -> ()
    n694 = Multiply(x=0.3 ("gyro scale"), y=w1002) -> (x*y=w589:dbl)
    "YR_FB" <- w589
    "Yawrate" <- w589
    n695 = Subtract(x=w972, y=w589) -> (x-y=w1026:dbl)
    n696 = feedback-in #32(w1026) -> ()
    n697 = formula code="float F,A,B,C,ykd,ykp,y0;\nF=2*tau+T;\nA=(2*Kd_rot)/F;\nB=(-2*Kd_rot)/F;\nC=(2*tau-T)/F;\nykd=A*u0+B*u1+C*y1;\nykp=Kp_rot*u0;\ny0=ykp+ykd;"("tau"=w1023, "u0"=w1026, "u1"=w1025, "y1"=w1030, "T"=0.001 ("input variable"), "Kp_rot"="Kp_rot 2", "Kd_rot"="Kd_rot 3") -> ("y0"=w1032:dbl)
    n698 = feedback-in #44(w1032) -> ()
    n699 = Select(t=w1032, s=w768, f=0.0) -> (s? t:f=w1038:dbl)
    n700 = Add(x=w974, y=w1038) -> (x+y=w1011:dbl)
    n701 = Bundle("Pmod_YR"=w1000, w1005, w1004, w1003, w589) -> (→"Gyro sensors":cluster{"Pmod_YR":dbl, dbl, dbl, dbl, dbl})  [unwired: 1 in]
    n702 = feedback-in #65(w589) -> ()
    n703 = formula code="float F,A,B,C,y0;\nF=2*tau+T;\nA=(2*a+b*T)/F;\nB=(b*T-2*a)/F;\nC=(2*tau-T)/F;\ny0=A*u0+B*u1+C*y1;"("tau"=w1056, "u0"=w589, "u1"=w1050, "y1"=w1049, "T"=w1051, "a"=w1048, "b"=w1047) -> ("y0"=w1039:dbl)
    n704 = feedback-in #75(w1039) -> ()
    n705 = Boolean To (0,1)(Boolean=w511) -> (0, 1=w870:i16)
    n706 = Boolean To (0,1)(Boolean=w511) -> (0, 1=w868:i16)
    n707 = Subtract(x=w1039, y=w1040) -> (x-y=w970:dbl)
    n708 = Boolean To (0,1)(Boolean=w511) -> (0, 1=w873:i16)
    n709 = Multiply(x=w873, y=w871) -> (x*y=w859:dbl)
    n710 = feedback #76(0.0) -> (w805:dbl)
    n711 = formula code="float F,A,B,C,y0;\nF=2*tau+T;\nA=(2*a+b*T)/F;\nB=(b*T-2*a)/F;\nC=(2*tau-T)/F;\ny0=A*u0+B*u1+C*y1;"("tau"=w800, "u0"=w801, "u1"=w807, "y1"=w805, "T"=0.001 ("입력 변수"), "a"=0.0 ("입력 변수"), "b"=1.0 ("입력 변수")) -> ("y0"=w682:dbl)
    n712 = feedback-in #76(w682) -> ()
    n713 = feedback #77(0.0) -> (w912:dbl)
    n714 = formula code="float F,A,B,C,y0;\nF=2*tau+T;\nA=(2*a+b*T)/F;\nB=(b*T-2*a)/F;\nC=(2*tau-T)/F;\ny0=A*u0+B*u1+C*y1;"("tau"=w800, "u0"=w798, "u1"=w914, "y1"=w912, "T"=0.001 ("입력 변수"), "a"=0.0 ("입력 변수"), "b"=1.0 ("입력 변수")) -> ("y0"=w721:dbl)
    n715 = feedback-in #77(w721) -> ()
    n716 = Multiply(x=w870, y=w869) -> (x*y=w860:dbl)
    n717 = Multiply(x=w868, y=w867) -> (x*y=w861:dbl)
    n718 = Boolean To (0,1)(Boolean=w481) -> (0, 1=w482:i16)
    n719 = feedback #78(0.0) -> (w812:dbl)
    n720 = formula code="float F,A,B,C,y0;\nF=2*tau+T;\nA=(2*a+b*T)/F;\nB=(b*T-2*a)/F;\nC=(2*tau-T)/F;\ny0=A*u0+B*u1+C*y1;"("tau"=w800, "u0"=w799, "u1"=w810, "y1"=w812, "T"=0.001 ("입력 변수"), "a"=0.0 ("입력 변수"), "b"=1.0 ("입력 변수")) -> ("y0"=w724:dbl)
    n721 = feedback-in #78(w724) -> ()
    n722 = Multiply(x=w482, y=i16 13) -> (x*y=w480:i16)
    n723 = formula code="int ASK;\n\nif (In2 ==2 && In8 ==0 && In13==0)\nASK = 2;\nelse if (In2 == 0 && In8 ==8 && In13==0)\nASK = 8;\nelse if (In2 == 0 && In8 ==0 && In13==13)\nASK = 13;\n\nelse if (SBCin == 4)\nASK = 9;\n\nelse \nASK =0;"("In2"=w663, "In8"=w662, "SBCin"=w543, "In13"=w480) -> ("ASK"=→"AskSBC":i32)
    n724 = Or(x=w370, y="FileCreat") -> (x .or. y?=w369:bool)
    n725 = Boolean To (0,1)(Boolean=w768) -> (0, 1=w1046:i16)
    n726 = Multiply(x=w1046, y=w970) -> (x*y=w1010:dbl)
    "YMO FB" <- w1010
    n727 = Subtract(x=w1011, y=w1010) -> (x-y=w819:dbl)
    n728 = Negate(x=w819) -> (-x=w824:dbl)
    n729 = feedback-in #56(w819) -> ()
    n730 = Select(t=w819, s=w823, f=w824) -> (s? t:f=w640:dbl)
    "AngCmdDOB" <- w640
    n731 = Add(x=w721, y=w640) -> (x+y=w683:dbl)
    "RearAngCmd" <- w683
    n732 = formula code="if (u >= lim*10/10)\ny0=lim*10/10;\nelse if (u <= -lim*10/10)\ny0=-lim*10/10;\nelse\ny0=u;"("u"=w861, "lim"="Tqlim") -> ("y0"=w630:dbl)
    n733 = formula code="if (u >= lim*10/10)\ny0=lim*10/10;\nelse if (u <= -lim*10/10)\ny0=-lim*10/10;\nelse\ny0=u;"("u"=w860, "lim"="Tqlim") -> ("y0"=w629:dbl)
    n734 = formula code="if (u >= lim*10/10)\ny0=lim*10/10;\nelse if (u <= -lim*10/10)\ny0=-lim*10/10;\nelse\ny0=u;"("u"=w859, "lim"="Tqlim") -> ("y0"=w863:dbl)
    n735 = local read "SBCSteerEnable"() -> (w764:bool)
    n736 = local read "SBCDriveEnable"() -> (w787:bool)
    n737 = feedback #79(0.0) -> (w383:dbl)
    n738 = case shown="참" w369 {
      tunnel: [w1168 w1169] -> w384
      tunnel: w383 -> [w1168 _]
      tunnel: w359 -> [_ w1169]
      frame False {
      }
      frame True {
      }
    }
    n739 = feedback-in #79(w384) -> ()
    n740 = formula code="if (u >= lim*10/10)\ny0=lim*10/10;\nelse if (u <= -lim*10/10)\ny0=-lim*10/10;\nelse\ny0=u;"("u"=w682, "lim"="Steeing_ang_limit") -> ("y0"=w625:dbl)
    "Tq_cmd_R" <- w625
    n741 = formula code="if (u >= lim*10/10)\ny0=lim*10/10;\nelse if (u <= -lim*10/10)\ny0=-lim*10/10;\nelse\ny0=u;"("u"=w724, "lim"="Steeing_ang_limit") -> ("y0"=w626:dbl)
    "Tq_cmd_L" <- w626
    n742 = formula code="if (u >= lim*10/10)\ny0=lim*10/10;\nelse if (u <= -lim*10/10)\ny0=-lim*10/10;\nelse\ny0=u;"("u"=w683, "lim"="Steeing_ang_limit") -> ("y0"=w627:dbl)
    "Tq_cmd_Rear" <- w627
    n743 = Subtract(x=w359, y=w384) -> (x-y=w372:dbl)
    n744 = Or(x=w787, y="DrivingEnable") -> (x .or. y?=w785:bool)
    n745 = Boolean To (0,1)(Boolean=w785) -> (0, 1=w1124:i16)
    n746 = Or(x="SteerEnable", y=w764) -> (x .or. y?=w779:bool)
    n747 = Boolean To (0,1)(Boolean=w779) -> (0, 1=w1122:i16)
    n748 = Greater?(x=w372, y=1.0) -> (0:w374:bool)
    n749 = Less?(x=w372, y=1.03) -> (x < y?=w373:bool)
    n750 = Multiply(x=w863, y="RearTqScale") -> (x*y=w628:dbl)
    n751 = Bundle("y0"=w630, "y0"=w629, w628) -> ()  [unwired: 1 in, 1 out]
    n752 = And(x=w374, y=w373) -> (x .and. y?=w371:bool)
    n753 = local write "Stop Button"(w371) -> ()
    n754 = Greater?(x=w372, y=0.0) -> (0:w380:bool)
    n755 = Less?(x=w372, y=0.03) -> (x < y?=w381:bool)
    n756 = And(x=w380, y=w381) -> (x .and. y?=w377:bool)
    n757 = local write "data iner"(w377) -> ()
    n758 = Multiply(x="Steer Enable", y=w1122) -> (x*y=w1127:fxp<+/-,36,21>)
    n759 = Multiply(x="Driving Enable", y=w1124) -> (x*y=w1128:fxp<+/-,36,21>)
    n760 = Negate(x=w628) -> (-x=w665:dbl)
    n761 = Negate(x=w629) -> (-x=w667:dbl)
    n762 = Negate(x=w630) -> (-x=w666:dbl)
    n763 = xnode "읽기/쓰기 컨트롤"("FPGA VI 참조 입력"=w1146, "에러 입력"=w1145, "Elmo1_Left"=w667, "Elmo2_Right"=w666, "Elmo3_Rear"=w665, "Elmo4_Steer_Left"=w625, "Elmo5_Steer_Right"=w626, "Elmo6_Steer_Rear"=w627, "Drive_enable"=w1128, "Steer_enable"=w1127) -> ()  [unwired: 2 out]
    n764 = node-c288() -> ()  [unwired: 1 in, 1 out]
    n765 = local read "Total_Stop"() -> (w1006:bool)
    "Time" <- w840
    "Tqoff_autoback" <- TRUE ("Tqoff_autoback")
  }
  n766 = while {
    tunnel: [w1294] -> _
    tunnel: [w1288] -> _
    tunnel: w6 -> [w1286]
    tunnel: w5 -> [w1285]
    i -> [w1287]
    stop <- w1284 stop-if-true
    w1290 = u32 4 ("바이트 카운트")
    n767 = property class="Instr"(reference=w1286, error in=w1285) -> (reference out=w1291:refnum<visa-resource-name>, error out=w1289:errorcluster, "Serial Settings:Number of Bytes at Serial Port"=w1293:u32)
    "버퍼된 문자개수" <- w1293
    n768 = Greater Or Equal?(x=w1293, y=w1290) -> (x >= y?=w1292:bool)
    n769 = case shown="참" w1292 {
      tunnel: [w1295 w1305] -> w1294
      tunnel: w1291 -> [w1295 w1304]
      tunnel: w1290 -> [_ w1301]
      tunnel: w1289 -> [w1296 w1303]
      tunnel: [w1296 w1297] -> w1288
      frame False {
      }
      frame True {
        n770 = VISA Read(VISA resource name=w1304, byte count=w1301, error in (no error)=w1303) -> (VISA resource name out=w1299:refnum<visa-resource-name>, read buffer=w1300:string, return count=w1302:u32, error out=w1298:errorcluster)
        n771 = Equal?(x=w1302, y=w1301) -> (x = y?=w1306:bool)
        n772 = case shown="참" w1306 {
          tunnel: w1300 -> [_ w1309]
          tunnel: [w1307 w1330] -> w1305
          tunnel: w1299 -> [w1307 w1326]
          tunnel: w1298 -> [w1308 w1325]
          tunnel: [w1308 w1324] -> w1297
          frame False {
          }
          frame True {
            n773 = flat-sequence {
              tunnel: w1309 -> [w1333]
              tunnel: [w1331] -> w1323
              tunnel: w1323 -> [w1343]
              tunnel: [w1344] -> w1322
              tunnel: [w1357] -> w1321
              tunnel: [w1356] -> w1320
              tunnel: w1322 -> [w1355]
              tunnel: [w1352] -> w1319
              tunnel: [w1351] -> w1318
              tunnel: w1321 -> [w1368]
              tunnel: [w1368] -> w1317
              tunnel: w1320 -> [w1367]
              tunnel: [w1367] -> w1316
              tunnel: w1319 -> [w1365]
              tunnel: w1318 -> [w1364]
              tunnel: [w1364] -> w1313
              tunnel: w1317 -> [w1379]
              tunnel: w1316 -> [w1377]
              tunnel: [w1381] -> w1310
              tunnel: [w1377] -> w1315
              tunnel: [w1376] -> w1311
              frame #0 {
                # "동기화 비트 추출"
                n774 = String To Byte Array(string=w1333) -> (unsigned byte array=w1332:u8[])
                n775 = for {
                  tunnel: w1332 -> [w1339] mode=indexing
                  tunnel: [w1335] -> w1331 mode=indexing
                  w1337 = 2  # 할당비트 수
                  w1338 = 5  # 동기화비트 인덱스
                  n776 = Number To Boolean Array(number=w1339) -> (Boolean array=w1334:bool[])
                  n777 = Array Subset(array=w1334, index=w1338, length=w1337) -> (w1336:bool[])
                  n778 = Boolean Array To Number(Boolean array=w1336) -> (number=w1335:u32)
                }
              }
              frame #1 {
                # "이전 동기화비트와 현재 동기화비트를 비교함\n이전 동기화비트에서 1을 더하여 현재와 비교함\n(동기화비트 3에서 1을 더할 경우\n4가 되므로 오류가 일어남 그래서\n동기화비트를 0으로 만듬)"
                n779 = feedback #80(w1343) -> (w1342:u32[])
                n780 = Increment(x=w1342) -> (x+1=w1341:u32[])
                n781 = feedback-in #80(w1343) -> ()
                n782 = for {
                  tunnel: [w1349] -> w1340 mode=indexing
                  tunnel: w1341 -> [w1346] mode=indexing
                  n783 = Greater?(x=w1346, y=u32 3 ("t")) -> (0:w1347:bool)
                  n784 = Select(t=u32 0, s=w1347, f=w1346) -> (s? t:f=w1349:u32)
                }
                n785 = Equal?(x=w1343, y=w1340) -> (x = y?=w1344:bool[])
              }
              frame #2 {
                n786 = feedback #81(u32[] [0, 0, 0, 0]) -> (w1353:u32[])
                n787 = for {
                  tunnel: w1353 -> [w1359] mode=indexing
                  tunnel: [w1360] -> w1352 mode=indexing
                  tunnel: w1355 -> [w1358] mode=indexing
                  # "동기화비트가 연속일 경우\n연속동기화회수를 증가"
                  n788 = case shown="참" w1358 {
                    tunnel: [u32 0 w1362] -> w1360
                    tunnel: w1359 -> [_ w1363]
                    frame False {
                    }
                    frame True {
                      n789 = Increment(x=w1363) -> (x+1=w1362:u32)
                    }
                  }
                }
                "인덱스별 첫번째 바이트일 연속동기화횟수 2" <- w1352
                n790 = feedback-in #81(w1352) -> ()
                n791 = Array Max & Min(array=w1352) -> (max value=w1351:u32, max index (indices)=w1356:i32)  [unwired: 2 out]
                n792 = Greater Or Equal?(x=w1351, y=u32 7 ("연속 동기화로 판단할 횟수 2")) -> (x >= y?=w1357:bool)
              }
              frame #3 {
                n793 = for {
                  tunnel: w1365 -> [w1375] mode=indexing
                  tunnel: w1364 -> [w1374]
                  tunnel: [w1369] -> w1366 mode=indexing
                  w1370 = 100.0  # %
                  n794 = To Double Precision Float(number=w1375) -> (double precision float=w1373:dbl)
                  n795 = To Double Precision Float(number=w1374) -> (double precision float=w1372:dbl)
                  n796 = Divide(x=w1373, y=w1372) -> (x/y=w1371:dbl)
                  n797 = Multiply(x=w1371, y=w1370) -> (x*y=w1369:dbl)
                }
                "인덱스별 첫번째 바이트일 확률(%) 2" <- w1366
              }
              frame #4 {
                # "연속 동기화로 판단되고(and)\n0번 바이트 동기화 되었을 경우\n동기화 완료"
                # "연속 동기화로 판단되고(and)\n0번 바이트 동기화 안 되었을 경우\n동기화가 필요"
                n798 = Equal To 0?(x=w1377) -> (x = 0?=w1378:bool)
                n799 = Compound Arithmetic op=AND ("복합 연산")(w1379, w1378) -> (w1376:bool)
                n800 = Not Equal To 0?(x=w1377) -> (x != 0?=w1380:bool)
                n801 = Compound Arithmetic op=AND ("복합 연산")(w1379, w1380) -> (w1381:bool)
              }
            }
            n802 = feedback #82(0) -> (w1328:i32)
            n803 = Increment(x=w1328) -> (x+1=w1327:i32)
            "현재 데이터 수신 횟수" <- w1327
            n804 = feedback-in #82(w1327) -> ()
            n805 = To Unsigned Long Integer(number=w1315) -> (unsigned 32bit integer=w1312:u32)
            n806 = case shown="참" w1311 {
              tunnel: w1309 -> [_ w1417]
              frame False {
              }
              frame True {
                n807 = String To Byte Array(string=w1417) -> (unsigned byte array=w1401:u8[])
                n808 = Index Array(array=w1401) -> (element #1=w1416:u8, element #2=w1412:u8, element #3=w1411:u8, element #4=w1410:u8)  [unwired: 4 in]
                n809 = Number To Boolean Array(number=w1416) -> (Boolean array=w1415:bool[])
                n810 = Index Array(array=w1415) -> (element #1=w1397:bool, element #2=w1395:bool, element #3=→"Parity":bool, element #4=w1405:bool, element #5=w1404:bool, element #6=w1407:bool, element #7=w1406:bool, element #8=→"Message Validity":bool)  [unwired: 8 in]
                n811 = Build Array(w1405, w1404) -> (w1414:bool[])
                n812 = Build Array(w1407, w1406) -> (w1402:bool[])
                n813 = Select(t=bool[] [TRUE, TRUE, TRUE, TRUE, TRUE, TRUE, TRUE, TRUE], s=w1395, f=bool[] [FALSE, FALSE, FALSE, FALSE, FALSE, FALSE, FALSE, FALSE]) -> (s? t:f=w1396:bool[])
                n814 = Number To Boolean Array(number=w1410) -> (Boolean array=w1398:bool[])
                n815 = Number To Boolean Array(number=w1411) -> (Boolean array=w1400:bool[])
                n816 = Number To Boolean Array(number=w1412) -> (Boolean array=w1399:bool[])
                n817 = Boolean Array To Number(Boolean array=w1414) -> (number=→"Type":u32)
                n818 = Boolean Array To Number(Boolean array=w1402) -> (number=→"Synchronization":u32)
                n819 = Build Array (concatenate)(w1398, w1400, w1399, w1397, w1395, w1396) -> (w1390:bool[])
                n820 = Boolean Array To Number(Boolean array=w1390) -> (number=w1392:u32)
                n821 = Split 1D Array(array=w1390, index=23) -> (first subarray=w1388:bool[], second subarray=w1383:bool[])
                "first subarray" <- w1388
                n822 = To Long Integer(number=w1392) -> (32bit integer=→"rawValue":i32)
                n823 = Index Array(array=w1383) -> (element=→"Direction(CW-T, CCW-F)":bool)  [unwired: 1 in]
                n824 = Boolean Array To Number(Boolean array=w1388) -> (number=w1387:u32)
                n825 = To Double Precision Float(number=w1387) -> (double precision float=w1385:dbl)
                n826 = Multiply(x=w1385, y=4.291534e-05) -> (x*y=→"OldAng":dbl)
              }
            }
            n827 = case shown="참" w1310 {
              tunnel: w1326 -> [w1419 w1427]
              tunnel: [w1419 w1426] -> w1330
              tunnel: w1312 -> [_ w1424]
              tunnel: w1327 -> [_ _]
              tunnel: w1325 -> [w1418 w1421]
              tunnel: [w1418 w1420] -> w1324
              frame False {
              }
              frame True {
                n828 = VISA Read(VISA resource name=w1427, byte count=w1424, error in (no error)=w1421) -> (VISA resource name out=w1426:refnum<visa-resource-name>, error out=w1420:errorcluster)  [unwired: 2 out]
                n829 = feedback #83(0) -> (w1430:i32)
                n830 = Increment(x=w1430) -> (x+1=w1429:i32)
                "데이터오류횟수" <- w1429
                n831 = feedback-in #83(w1429) -> ()
                n832 = feedback #84(u32[] []) -> (w1423:u32[])
                n833 = Build Array (concatenate)(w1423, w1424) -> (w1422:u32[])
                "동기화된 인덱스번호" <- w1422
                n834 = feedback-in #84(w1422) -> ()
              }
            }
            "최대 연속 동기화 횟수" <- w1313
            "현재 동기화 완료" <- w1311
            "error out 2" <- "error in 2"
          }
        }
      }
    }
    n835 = local read "Total_Stop"() -> (w1284:bool)
    "datameasure" <- w1287
  }
  n836 = Merge Errors(w27, w26) -> (w25:errorcluster)
  n837 = xnode "Close FPGA VI Reference"("FPGA VI 참조 입력"=w31, "에러 입력"=w25) -> ("에러 출력"=w52:errorcluster)
  n838 = call <vilib>:"Simple Error Handler.vi"("error in (no error)"=w52) -> ("error out"=w28:errorcluster)  [unwired: 4 in, 4 out]
  n839 = flat-sequence {
    tunnel: w28 -> [_]
    frame #0 {
      n840 = local write "Total_Stop"(FALSE ("정지")) -> ()
    }
  }
  n841 = node-c288(w29) -> ()  [unwired: 1 out]
  n842 = while {
    i -> [w1442]
    stop <- "file create" stop-if-true
    n843 = Format Date/Time String(time format string (%c)="%Y%m%d_%H%M%S%3u") -> (date/time string=w1440:string)  [unwired: 2 in]
    n844 = Strip Path(path=path "U:/exp") -> (stripped path=w1435:path)  [unwired: 1 out]
    n845 = Concatenate Strings(w1440, ".csv" ("string")) -> (w1438:string)
    n846 = Build Path(base path=w1435, name or relative path=w1438) -> (appended path=w1437:path)
    n847 = while {
      i -> [w1475]
      stop <- "Stop Button" stop-if-true
      "Numeric Control" <- w1475
    }
    n848 = Open/Create/Replace File(file path (use dialog)=w1437, operation (0:open)=T15."create") -> (refnum out=w1433:refnum<file>)  [unwired: 4 in, 2 out]
    n849 = while {
      tunnel: w1433 -> [w1466]
      tunnel: [w1465] -> w1432
      i -> [w1474]
      stop <- "data iner" stop-if-true
      n850 = Wait Until Next ms Multiple(millisecond multiple=u32 10 ("ms 배수")) -> ()  [unwired: 1 out]
      n851 = local read "SendDataOn"() -> (w1457:bool)
      n852 = local read "SinTx"() -> (w1448:dbl)
      n853 = local read "AskSBC"() -> (w1451:i16)
      n854 = local read "Jm_rot"() -> (w1447:dbl)
      n855 = local read "SBCmode 2"() -> (w1444:dbl)
      n856 = Boolean To (0,1)(Boolean=w1457) -> (0, 1=w1455:i16)
      n857 = local read "Vel_Robot"() -> (w1461:dbl)
      n858 = local read "SBCmode"() -> (w1454:dbl)
      n859 = local read "NowAng"() -> (w1458:dbl)
      n860 = Format Date/Time String(time format string (%c)="%H%M%S%3u") -> (date/time string=w1470:string)  [unwired: 2 in]
      n861 = local read "AngRer"() -> (w1459:dbl)
      n862 = local read "x_Rear"() -> (w1462:dbl)
      n863 = local read "VelRef"() -> (w1460:dbl)
      n864 = local read "x_L"() -> (w1449:dbl)
      n865 = local read "x_R"() -> (w1463:dbl)
      n866 = Multiply(x=w1451, y=1.0) -> (x*y=w1450:dbl)
      n867 = Multiply(x=w1455, y=1.0) -> (x*y=w1453:dbl)
      n868 = Bundle("x_L"=w1449, "x_R"=w1463, "x_Rear"=w1462, "Vel_Robot"=w1461, "VelRef"=w1460, "AngRer"=w1459, "NowAng"=w1458, w1450, "SBCmode"=w1454, "SinTx"=w1448, "Jm_rot"=w1447, w1453, "SBCmode 2"=w1444) -> (w1446:T16)  [unwired: 1 in]
      n869 = Cluster To Array(cluster=w1446) -> (array=w1445:dbl[])
      n870 = Array To Spreadsheet String(array=w1445, 3:"%f" ("format string")) -> (spreadsheet string=w1467:string)  [unwired: 1 in]
      n871 = Concatenate Strings(w1470, "\t", w1467) -> (w1472:string)
      n872 = Write to Text File(file (use dialog)=w1466, text=w1472) -> (refnum out=w1465:refnum<file>)  [unwired: 2 in, 2 out]
      "data innter" <- w1474
    }
    n873 = Close File(refnum=w1432) -> ()  [unwired: 1 in, 2 out]
    "File create" <- w1442
  }
